vi "Global_SNK3_HF.vi"() -> ()   [LabVIEW 2017]
uses:
  Control_EU/UNDT_ClusterPackRevers (Type).ctl
  Control_EU/OptionPACK5.ctl
  E:/_git/LV_Unicorn/Control/unicorn_Param.ctl
  E:/_git/LV_Unicorn/Control/unicorn_conn.ctl
  E:/_git/LV_Unicorn/Control/unicorn_JSON.ctl
  E:/_git/LV_Unicorn/Control/unicorn_ParamInt.ctl
  E:/_git/LV_Unicorn/Control/unicorn_Telemetry.ctl
  E:/_git/LV_Unicorn/Control/unicorn_Table.ctl
  E:/_git/LV_Unicorn/Control/unicorn_ParamFloat.ctl
  E:/_git/LV_Unicorn/Control/AnswerUDP.ctl
  Control_EU/MeasControl.ctl
  E:/_git/LV_Unicorn/LV_Unicorn.lvlib
panel:
  in  "Tab Control":T1(tab)
  out "UDP1_packet_size":u16=652 caption="UDP0_packet_size"
  out "UDP1_packet_speed":dbl=652.0 caption="UDP1 packet size [Mbit/s]"
  out "UDP0_packet_speed":dbl=652.0 caption="UDP0 packet size [Mbit/s]"
  out "UDP0_EnquOverflow":bool
  out "UDP1_EnquOverflow":bool
  out "UDP0_total_size":u16=652 caption="UDP0_packet_size"
  out "UDP1_packet_nuber":u32=1995311 caption="UDP0_packet_nuber"
  out "UDP1_LostPack":u32 caption="UDP0__lost_pack"
  out "UDP1_iter_cnt":i32=7055 caption="UDP0_iter_count"
  in  "IndEnqu":enum16{"NoEnqu", "LossyEnqu", "Enqu"}(ring)=enum."Enqu"
  in  "LossyEnq":bool=TRUE
  out "UDP0":string
  out "UDP0_PackEnd_bad":u32
  out "UDP0_CRC8_bad":u32
  out "UDP0_LostPack":u32 caption="UDP0__lost_pack"
  out "UDP0_packet_size":u16=652
  out "UDP0_packet_nuber":u32=1995311
  out "UDP0_length":i32=2052
  out "UDP0_Reserv":u8
  out "UDP0_offset":i32
  out "UDP0_AscanLostPack":u32
  out "UDP0_address":u32=3232235999 format="%x"
  out "UDP0_port":u16=1555
  out "UDP0_timeout":i32=1000
  out "UDP0_iter_count":i32=7055
  in  "UDP_buf_size":i32=4000000
  in  "rx_port_0":u16=1556 caption="Порт приемника 2"
  in  "rx_port_1":u16=1557 caption="Порт приемника 1"
  in  "#UDP_pack":u32=1 min=1 max=100
  out "#el_queue":i32
  out "UNDT_Cl1":T2={"PacketCounter"=998360, "Gain Coeff"=0.0, "SamplingInterval"=2e-08, "Lose Packet"=8, "EncodersParam2"=0, "EncodersParam1"=0, "Reserve 1"=0, "Mux TX/RX"=0, "ScanDelay"=0, "CRC 8"=86, "ScanDuration"=500, "N chanel"=0, "GlobalTime2"=63660000, "GlobalTime1"=11423, "N tick"=0, "Ncycle"=15329, "FrameFormatVersion"=1, "MagicWord"=305419896, "Overload"=FALSE} {"Gain Coeff" format="%_5e"; "Reserve 1" format="%02x"; "Mux TX/RX" format="%02x"; "ScanDelay" format="%02x"; "SamplingInterval" format="%_3e"; "Lose Packet" format="%08x"; "EncodersParam2" format="%016x"; "EncodersParam1" format="%016x"; "CRC 8" format="%02x"; "N chanel" format="%02x"; "N tick" format="%02x"; "FrameFormatVersion" format="%02x"; "MagicWord" format="%.0x"}
  out "UNDT_Cl0":T2={"PacketCounter"=998360, "Gain Coeff"=0.0, "SamplingInterval"=2e-08, "Lose Packet"=8, "EncodersParam2"=0, "EncodersParam1"=0, "Reserve 1"=0, "Mux TX/RX"=0, "ScanDelay"=0, "CRC 8"=86, "ScanDuration"=500, "N chanel"=0, "GlobalTime2"=63660000, "GlobalTime1"=11423, "N tick"=0, "Ncycle"=15329, "FrameFormatVersion"=1, "MagicWord"=305419896, "Overload"=FALSE} {"Gain Coeff" format="%_5e"; "Reserve 1" format="%02x"; "Mux TX/RX" format="%02x"; "ScanDelay" format="%02x"; "SamplingInterval" format="%_3e"; "Lose Packet" format="%08x"; "EncodersParam2" format="%016x"; "EncodersParam1" format="%016x"; "CRC 8" format="%02x"; "N chanel" format="%02x"; "N tick" format="%02x"; "FrameFormatVersion" format="%02x"; "MagicWord" format="%.0x"}
  in  "UDP0_EnbLog":bool
  in  "SUdpAnswer":T3
  in  "paramUnicorn":T4={"conParam"={"ReadIntParam"=TRUE, "ReadDescrParam"=FALSE, "ReadFloatParam"=TRUE, "debug"=FALSE, "ReadJSON"=TRUE, "IP_address"="192.168.1.216", "N_attempts"=3, "type_con"=enum."TCP", "MB_address"=1, "VISA"="COM1", "connection ID"=refnum, "nameDevices"="", "timeout"=500, "port"=2000, "type_version"="0F0C0001", "baud_rate"=115200, "VersionControl"=TRUE, "TCP_conn"=FALSE, "WindowSize"=400}, "Param"={"NumParam"={"NTelem"=201, "NInt"=16, "NFloat"=10, "NTable"=2}, "ParamInt"=[], "Telemetry"=[], "Table"=[], "ParamFloat"=[]}}
  in  "reqTypeVer":i32=252444676 format="%08x"
  out "IP_PC":string="192.168.1.99" caption="IP адрес ПК"
  out "JSONStr":string="{ \"UUID\": true, \"Reset\": false, \"Enums\": [ { \"ID\": \"Enum_AlarmCompMode\", \"Name\": \"Alarm comparison mode\", \"Desc\": \"\", \"Values\": [ { \"Name\": \"XY\", \"Value\": 0, \"Desc\": \"Available for rectangular and sector zones\" }, { \"Name\": \"AT\", \"Value\": 1, \"Desc\": \"Available for measurement zone\" }, { \"Name\": \"XT\", \"Value\": 2, \"Desc\": \"Available for measurement zone\" }, { \"Name\": \"YT\", \"Value\": 3, \"Desc\": \"Available for measurement zone\" } ] }, { \"ID\": \"Enum_AlarmZonesMode\", \"Name\": \"Alarm zones mode\", \"Desc\": \"\", \"Values\": [ { \"Name\": \"off\", \"Value\": 0, \"Desc\": \"\" }, { \"Name\": \"Rectangle\", \"Value\": 1, \"Desc\": \"\" }, { \"Name\": \"sector\", \"Value\": 2, \"Desc\": \"\" }, { \"Name\": \"measurement\", \"Value\": 3, \"Desc\": \"\" } ] }, { \"ID\": \"Enum_AlarmLEDMode\", \"Name\": \"Alarm LED mode\", \"Desc\": \"\", \"Values\": [ { \"Name\": \"off\", \"Value\": 0, \"Desc\": \"LED is always off\" }, { \"Name\": \"On\", \"Value\": 1, \"Desc\": \"LED is always on\" }, { \"Name\": \"Zone1\", \"Value\": 2, \"Desc\": \"LED is on if zone 1\" }, { \"Name\": \"Zone2\", \"Value\": 3, \"Desc\": \"LED is on if zone 2\" }, { \"Name\": \"Zone3\", \"Value\": 4, \"Desc\": \"LED is on if zone 3\" }, { \"Name\": \"Zone12\", \"Value\": 5, \"Desc\": \"LED is on if zone 1 or 2\" }, { \"Name\": \"Zone13\", \"Value\": 6, \"Desc\": \"LED is on if zone 1 or 3\" }, { \"Name\": \"Zone23\", \"Value\": 7, \"Desc\": \"LED is on if zone 2 or 3\" }, { \"Name\": \"Zone123\", \"Value\": 8, \"Desc\": \"LED is on if zone 1 or 2 or 3\" } ] }, { \"ID\": \"Enum_ModeWork\", \"Name\": \"Device operation mode\", \"Desc\": \"\", \"Values\": [ { \"Name\": \"Ошибка\", \"Value\": -1, \"Desc\": \"\" }, { \"Name\": \"Конфигурирование\", \"Value\": 0, \"Desc\": \"\" }, { \"Name\": \"Сканирование\", \"Value\": 1, \"Desc\": \"\" }, { \"Name\": \"Самотестирование\", \"Value\": 2, \"Desc\": \"\" } ] }, { \"ID\": \"OnOffEnum\", \"Name\": \"On-off enum\", \"Num\": 0, \"Values\": [ { \"Name\": \"Выключено\", \"Value\": 0 }, { \"Name\": \"Включено\", \"Value\": 1 } ] }, { \"ID\": \"InvNoInvEnum\", \"Name\": \"Invert-Noinvert enum\", \"Num\": 0, \"Values\": [ { \"Name\": \"Не инвертирован\", \"Value\": 0 }, { \"Name\": \"Интерирован\", \"Value\": 1 } ] }, { \"ID\": \"Enum_SyncMode\", \"Name\": \"Режим работы узла синхронизации \", \"Desc\": \"\", \"Values\": [ { \"Name\": \"Таймер\", \"Value\": 1, \"Desc\": \"\" }, { \"Name\": \"Энкодер\", \"Value\": 2, \"Desc\": \"\" }, { \"Name\": \"Импульс\", \"Value\": 3, \"Desc\": \"\" } ] }, { \"ID\": \"Enum_LPFilter\", \"Name\": \"ФНЧ приемников\", \"Desc\": \"\", \"Values\": [ { \"Name\": \"14\", \"Value\": 0, \"Desc\": \"\" }, { \"Name\": \"10\", \"Value\": 1, \"Desc\": \"\" }, { \"Name\": \"7,5\", \"Value\": 2, \"Desc\": \"\" }, { \"Name\": \"Выключен\", \"Value\": 3, \"Desc\": \"\" } ] }, { \"ID\": \"Enum_HPFilter\", \"Name\": \"ФВЧ приемников\", \"Desc\": \"\", \"Values\": [ { \"Name\": \"Выключен\", \"Value\": 0, \"Desc\": \"\" }, { \"Name\": \"1\", \"Value\": 1, \"Desc\": \"\" }, { \"Name\": \"2\", \"Value\": 2, \"Desc\": \"\" } ] }, { \"ID\": \"Enum_PatternMode\", \"Name\": \"Тестирование цифрового интерфейса АЦП\", \"Desc\": \"\", \"Values\": [ { \"Name\": \"No pattern\", \"Value\": 0, \"Desc\": \"\" }, { \"Name\": \"Sync\", \"Value\": 1, \"Desc\": \"\" }, { \"Name\": \"Deskew\", \"Value\": 2, \"Desc\": \"\" }, { \"Name\": \"Custom\", \"Value\": 3, \"Desc\": \"\" }, { \"Name\": \"All 1s\", \"Value\": 4, \"Desc\": \"\" }, { \"Name\": \"Toggle\", \"Value\": 5, \"Desc\": \"\" }, { \"Name\": \"All 0s\", \"Value\": 6, \"Desc\": \"\" }, { \"Name\": \"Ramp\", \"Value\": 7, \"Desc\": \"\" } ] }, { \"ID\": \"Enum_PulserLevel\", \"Name\": \"Амплитуда импульсов возбуждения ГИ\", \"Desc\": \"\", \"Values\": [ { \"Name\": \"20\", \"Value\": 0, \"Desc\": \"\" }, { \"Name\": \"40\", \"Value\": 1, \"Desc\": \"\" }, { \"Name\": \"60\", \"Value\": 2, \"Desc\": \"\" }, { \"Name\": \"80\", \"Value\": 3, \"Desc\": \"\" }, { \"Name\": \"100\", \"Value\": 4, \"Desc\": \"\" }, { \"Name\": \"120\", \"Value\": 5, \"Desc\": \"\" }, { \"Name\": \"140\", \"Value\": 6, \"Desc\": \"\" }, { \"Name\": \"160\", \"Value\": 7, \"Desc\": \"\" }, { \"Name\": \"180\", \"Value\": 8, \"Desc\": \"\" }, { \"Name\": \"200\", \"Value\": 9, \"Desc\": \"\" } ] }, { \"ID\": \"DACParamEnum\", \"Name\": \"Параметр, определяющий коэффициента усиления приемников \", \"Values\": [ { \"Name\": \"Коэф. усил. (дБ)\", \"Value\": 0 }, { \"Name\": \"Вых. ЦАП (10 бит)\", \"Value\": 1 }, { \"Name\": \"Вых. ЦАП (8 бит)\", \"Value\": 1 } ] } ], \"ParamInt\": [ { \"ID\": \"ModeWork\", \"Num\": 0, \"Name\": \"Режим работы\", \"Type\": \"enum\", \"Enum\": \"Enum_ModeWork\", \"Desc\": \"\", \"Unit\": \"\", \"Access\": \"ro\" }, { \"ID\": \"CCEnable\", \"Num\": 1, \"Name\": \"Режим сканирования\", \"Type\": \"enum\", \"Enum\": \"OnOffEnum\", \"Desc\": \"Включение режима выполнения циклов сканирования\", \"Unit\": \"\", \"Access\": \"rw\" }, { \"ID\": \"CCTicksCount\", \"Num\": 2, \"Name\": \"Количество тактов\", \"Type\": \"Regular\", \"Desc\": \"Количество тактов выполняемых в каждом цикле при включении режима сканирования\", \"Unit\": \"\", \"Min\": 1, \"Max\": 32, \"FormatStr\": \"%d\", \"Access\": \"rw\" }, { \"ID\": \"LPFilter\", \"Num\": 3, \"Name\": \"ФНЧ приемников\", \"Type\": \"enum\", \"Enum\": \"Enum_LPFilter\", \"Desc\": \"Частота среза фильтра низких частот приемников сигналов элементов ФЛ\", \"Unit\": \"МГц\", \"Access\": \"rw\" }, { \"ID\": \"HPFilter\", \"Num\": 4, \"Name\": \"ФВЧ приемников\", \"Type\": \"Regular\", \"Min\": 0, \"Max\": 10, \"FormatStr\": \"%d\", \"Desc\": \"Параметр определяющий частоту среза фильтра высоких частот приемников сигналов элементов ФЛ \", \"Unit\": \"\", \"Access\": \"rw\" }, { \"ID\": \"TestTickNum\", \"Num\": 5, \"Name\": \"Номер такта для тестового захвата\", \"Desc\": \"Номер такта для выполнения тестирования настроек выбранного такта \", \"Unit\": \"\", \"Min\": 1, \"Max\": 32, \"FormatStr\": \"%d\", \"Access\": \"rw\" }, { \"ID\": \"Pulser1Level\", \"Num\": 6, \"Name\": \"Амплитуда импульсов возбуждения ГИ №1 для каналов 1…8\", \"Type\": \"enum\", \"Enum\": \"Enum_PulserLevel\", \"Desc\": \"Амплитуда импульсов возбуждения для ПЭП с 1 по 8\", \"Unit\": \"В\", \"Access\": \"rw\" }, { \"ID\": \"Pulser2Level\", \"Num\": 7, \"Name\": \"Амплитуда импульсов возбуждения ГИ №2 для каналов 9…16\", \"Type\": \"enum\", \"Enum\": \"Enum_PulserLevel\", \"Desc\": \"Амплитуда импульсов возбуждения для ПЭП с 9 по 16\", \"Unit\": \"В\", \"Access\": \"rw\" }, { \"ID\": \"IPDefaultAddress\", \"Num\": 8, \"Name\": \"IP адрес электронного блока по умолчанию\", \"Type\": \"IPv4Addr\", \"Desc\": \"Присваивается электронному блоку если не был получен автоматически от DCHP сервера\", \"Unit\": \"IPv4\", \"Access\": \"rw\" }, { \"ID\": \"IPDefaultNetMask\", \"Num\": 9, \"Name\": \"Маска подсети\", \"Type\": \"IPv4Mask\", \"Desc\": \"Присваивается электронному блоку если не был получен автоматически от DCHP сервера\", \"Unit\": \"IPv4\", \"Access\": \"rw\" }, { \"ID\": \"IPDefaultGW\", \"Num\": 10, \"Name\": \"Основной шлюз \", \"Type\": \"IPv4Addr\", \"Desc\": \"Присваивается электронному блоку если не был получен автоматически от DCHP сервера\", \"Unit\": \"IPv4\", \"Access\": \"rw\" }, { \"ID\": \"IPCurrentAddress\", \"Num\": 11, \"Name\": \"Текущий IP адрес электронного блока\", \"Type\": \"IPv4Addr\", \"Desc\": \"Присваивается электронному блоку DCHP сервером\", \"Unit\": \"IPv4\", \"Access\": \"ro\" }, { \"ID\": \"IPAddressUDP\", \"Num\": 12, \"Name\": \"IP адрес для передачи UDP пакетов\", \"Type\": \"IPv4Addr\", \"Desc\": \"IP адрес на который будут отправляется информационные UDP пакеты\", \"Unit\": \"IPv4\", \"Access\": \"rw\" }, { \"ID\": \"Port1UDP\", \"Num\": 13, \"Name\": \"Порт для передачи UDP пакетов от ГИ №1, каналы 1…8\", \"Type\": \"Regular\", \"Desc\": \"Порт, на который будут отправляется информационные UDP пакеты от ГИ №1, каналы 1…8\", \"Unit\": \"\", \"Min\": 0, \"Max\": 65535, \"FormatStr\": \"%d\", \"Access\": \"rw\" }, { \"ID\": \"Port2UDP\", \"Num\": 14, \"Name\": \"Порт для передачи UDP пакетов от ГИ №2, каналы 9…16\", \"Type\": \"Regular\", \"Desc\": \"Порт, на который будут отправляется информационные UDP пакеты от ГИ №2, каналы 9…16\", \"Unit\": \"\", \"Min\": 0, \"Max\": 65535, \"FormatStr\": \"%d\", \"Access\": \"rw\" }, { \"ID\": \"IPFPGA1TypeVer\", \"Num\": 15, \"Name\": \"Тип и версия ПЛИС №1\", \"Type\": \"Regular\", \"Desc\": \"Тип и версия встроенного ПО ПЛИС платы приема\", \"Unit\": \"\", \"FormatStr\": \"0x%08x\", \"Access\": \"ro\" }, { \"ID\": \"IPFPGA1BuildTime\", \"Num\": 16, \"Name\": \"Дата сборки ПО ПЛИС №1\", \"Type\": \"DateTime\", \"Desc\": \"Дата сборки встроенного ПО ПЛИС платы приема\", \"Unit\": \"\", \"FormatStr\": \"%T\", \"Access\": \"ro\" }, { \"ID\": \"IPFPGA2TypeVer\", \"Num\": 17, \"Name\": \"Тип и версия ПЛИС №2\", \"Type\": \"Regular\", \"Desc\": \"Тип и версия встроенного ПО ПЛИС платы приема\", \"Unit\": \"\", \"FormatStr\": \"0x%08x\", \"Access\": \"ro\" }, { \"ID\": \"IPFPGA2BuildTime\", \"Num\": 18, \"Name\": \"Дата сборки ПО ПЛИС №2\", \"Type\": \"DateTime\", \"Desc\": \"Дата сборки встроенного ПО ПЛИС платы приема\", \"Unit\": \"\", \"FormatStr\": \"%T\", \"Access\": \"ro\" }, { \"ID\": \"IPADCMonMCUBuildTime\", \"Num\": 19, \"Name\": \"Дата сборки ПО МК мониторинга\", \"Type\": \"DateTime\", \"Desc\": \"Дата сборки ПО МК мониторинга платы приема\", \"Unit\": \"\", \"FormatStr\": \"%T\", \"Access\": \"ro\" }, { \"ID\": \"IPPMD2MCUBuildTime\", \"Num\": 20, \"Name\": \"Дата сборки ПО МК мониторинга ИП D2\", \"Type\": \"DateTime\", \"Desc\": \"Дата сборки ПО МК мониторинга платы источника питания D2\", \"Unit\": \"\", \"FormatStr\": \"%T\", \"Access\": \"ro\" }, { \"ID\": \"IPPMD4MCUBuildTime\", \"Num\": 21, \"Name\": \"Дата сборки ПО МК мониторинга ИП D6\", \"Type\": \"DateTime\", \"Desc\": \"Дата сборки ПО МК мониторинга платы источника питания D6\", \"Unit\": \"\", \"FormatStr\": \"%T\", \"Access\": \"ro\" }, { \"ID\": \"IPSaveParem\", \"Num\": 22, \"Name\": \"Сохранение параметров\", \"Type\": \"bool\", \"Desc\": \"Сохранение параметров в энергонезависимую память\", \"Unit\": \"\", \"FormatStr\": \"\", \"Access\": \"rw\" }, { \"ID\": \"IPSyncMode\", \"Num\": 23, \"Name\": \"Режим работы узла синхронизации \", \"Type\": \"enum\", \"Enum\": \"Enum_SyncMode\", \"Desc\": \"Режим работы узла синхронизации \", \"Access\": \"rw\" }, { \"ID\": \"IPTimerSyncInt\", \"Num\": 24, \"Name\": \"Интервал времени запуска выполнения цикла в режиме «Таймер»\", \"Type\": \"Regular\", \"Desc\": \"-\", \"Unit\": \"мкс\", \"Min\": 1000, \"Max\": 1000000, \"FormatStr\": \"%d\", \"Access\": \"rw\" }, { \"ID\": \"IPEncoder2En\", \"Num\": 25, \"Name\": \"Разрешение работы энкодера 2\", \"Type\": \"enum\", \"Desc\": \"\", \"Enum\": \"OnOffEnum\", \"Access\": \"rw\" }, { \"ID\": \"IPEncoder1En\", \"Num\": 26, \"Name\": \"Разрешение работы энкодера 1\", \"Type\": \"enum\", \"Desc\": \"\", \"Enum\": \"OnOffEnum\", \"Access\": \"rw\" }, { \"ID\": \"IPEncoderNum\", \"Num\": 27, \"Name\": \"Номер энкодера для режима «Энкодер»\", \"Type\": \"Regular\", \"Desc\": \"\", \"Unit\": \"\", \"Min\": 1, \"Max\": 2, \"FormatStr\": \"%d\", \"Access\": \"rw\" }, { \"ID\": \"IPEncoder2ZEn\", \"Num\": 28, \"Name\": \"Энкорер 2 разрешение сброса по сигналу «Z»\", \"Type\": \"enum\", \"Desc\": \"\", \"Enum\": \"OnOffEnum\", \"Access\": \"rw\" }, { \"ID\": \"IPEncoder2ZInv\", \"Num\": 29, \"Name\": \"Энкорер 2 инверсия сигнала «Z»\", \"Type\": \"enum\", \"Desc\": \"\", \"Enum\": \"OnOffEnum\", \"Access\": \"rw\" }, { \"ID\": \"IPEncoder2BInv\", \"Num\": 30, \"Name\": \"Энкорер 2 инверсия сигнала «B»\", \"Type\": \"enum\", \"Desc\": \"\", \"Enum\": \"OnOffEnum\", \"Access\": \"rw\" }, { \"ID\": \"IPEncoder2AInv\", \"Num\": 31, \"Name\": \"Энкорер 2 инверсия сигнала «A»\", \"Type\": \"enum\", \"Desc\": \"\", \"Enum\": \"OnOffEnum\", \"Access\": \"rw\" }, { \"ID\": \"IPEncoder1ZEn\", \"Num\": 32, \"Name\": \"Энкорер 1 разрешение сброса по сигналу «Z»\", \"Type\": \"enum\", \"Desc\": \"\", \"Enum\": \"OnOffEnum\", \"Access\": \"rw\" }, { \"ID\": \"IPEncoder1ZInv\", \"Num\": 33, \"Name\": \"Энкорер 1 инверсия сигнала «Z»\", \"Type\": \"enum\", \"Desc\": \"\", \"Enum\": \"OnOffEnum\", \"Access\": \"rw\" }, { \"ID\": \"IPEncoder1BInv\", \"Num\": 34, \"Name\": \"Энкорер 1 инверсия сигнала «B»\", \"Type\": \"enum\", \"Desc\": \"\", \"Enum\": \"OnOffEnum\", \"Access\": \"rw\" }, { \"ID\": \"IPEncoder1AInv\", \"Num\": 35, \"Name\": \"Энкорер 1 инверсия сигнала «A»\", \"Type\": \"enum\", \"Desc\": \"\", \"Enum\": \"OnOffEnum\", \"Access\": \"rw\" }, { \"ID\": \"IPPulseCounterEn\", \"Num\": 36, \"Name\": \"Разрешение работы счетчика импульсов \", \"Type\": \"enum\", \"Desc\": \"\", \"Enum\": \"OnOffEnum\", \"Access\": \"rw\" }, { \"ID\": \"IPPulseInput\", \"Num\": 37, \"Name\": \"Вход импульса запуска для режима «Импульс»\", \"Type\": \"enum\", \"Desc\": \"\", \"Enum\": { \"ID\": \"IPPulseInputEnum\", \"Values\": [ { \"Desc\": \"Использовать сигнал со входа SY1_DIN1\", \"Name\": \"SY1_DIN1\", \"Value\": 0 }, { \"Desc\": \"Использовать сигнал со входа SY1_DIN2\", \"Name\": \"SY1_DIN2\", \"Value\": 1 }, { \"Desc\": \"Использовать сигнал со входа SY1_DIN3\", \"Name\": \"SY1_DIN3\", \"Value\": 2 }, { \"Desc\": \"Использовать сигнал со входа SY1_DIN4\", \"Name\": \"SY1_DIN4\", \"Value\": 3 }, { \"Desc\": \"Использовать сигнал со входа SY1_DIN5\", \"Name\": \"SY1_DIN5\", \"Value\": 4 }, { \"Desc\": \"Использовать сигнал со входа SY1_DIN6\", \"Name\": \"SY1_DIN6\", \"Value\": 5 } ] }, \"Access\": \"rw\" }, { \"ID\": \"IPPulseSensitivity\", \"Num\": 38, \"Name\": \"Чувствительность входа импульсов\", \"Type\": \"enum\", \"Desc\": \"\", \"Enum\": { \"ID\": \"IPPulseSensitivityEnum\", \"Values\": [ { \"Desc\": \"Резерв, счетчик не работает\", \"Name\": \"Резерв\", \"Value\": 0 }, { \"Desc\": \"по фронту импульса\", \"Name\": \"Фронт\", \"Value\": 1 }, { \"Desc\": \"по срезу импульса\", \"Name\": \"Срез\", \"Value\": 2 }, { \"Desc\": \"и по фронту и по срезу импульса\", \"Name\": \"Оба\", \"Value\": 3 } ] }, \"Access\": \"rw\" }, { \"ID\": \"IPDataEncodersParam2\", \"Num\": 39, \"Name\": \"Параметры поля «EncodersParam2»\", \"Type\": \"enum\", \"Desc\": \"\", \"Enum\": { \"ID\": \"IPDataEncodersParam2Enum\", \"Values\": [ { \"Desc\": \"Текущее значение счетчика энкодера 2\", \"Name\": \"Encoder2CurrData\", \"Value\": 0 }, { \"Desc\": \"Текущее значение счетчика импульсов\", \"Name\": \"PulseCurrData\", \"Value\": 1 } ] }, \"Access\": \"rw\" }, { \"ID\": \"IPDataEncodersParam1\", \"Num\": 40, \"Name\": \"Параметры поля «EncodersParam1»\", \"Type\": \"enum\", \"Desc\": \"\", \"Enum\": { \"ID\": \"IPDataEncodersParam1Enum\", \"Values\": [ { \"Desc\": \"Текущее значение счетчика энкодера 1\", \"Name\": \"Encoder1CurrData\", \"Value\": 0 }, { \"Desc\": \"Текущее значение счетчика импульсов\", \"Name\": \"PulseCurrData\", \"Value\": 1 } ] }, \"Access\": \"rw\" }, { \"ID\": \"IPEncoder1CurrDataH\", \"Num\": 41, \"Name\": \"Текущее значение счетчика энкодера 1 [старшие 32 разряда]\", \"Type\": \"Regular\", \"Desc\": \"\", \"Unit\": \"\", \"FormatStr\": \"0x%08x\", \"Access\": \"rw\" }, { \"ID\": \"IPEncoder1CurrDataL\", \"Num\": 42, \"Name\": \"Текущее значение счетчика энкодера 1 [младшие 32 разряда]\", \"Type\": \"Regular\", \"Desc\": \"\", \"Unit\": \"\", \"FormatStr\": \"0x%08x\", \"Access\": \"rw\" }, { \"ID\": \"IPEncoder2CurrDataH\", \"Num\": 43, \"Name\": \"Текущее значение счетчика энкодера 2 [старшие 32 разряда]\", \"Type\": \"Regular\", \"Desc\": \"\", \"Unit\": \"\", \"FormatStr\": \"0x%08x\", \"Access\": \"rw\" }, { \"ID\": \"IPEncoder2CurrDataL\", \"Num\": 44, \"Name\": \"Текущее значение счетчика энкодера 2 [младшие 32 разряда]\", \"Type\": \"Regular\", \"Desc\": \"\", \"Unit\": \"\", \"FormatStr\": \"0x%08x\", \"Access\": \"rw\" }, { \"ID\": \"IPPulseCurrDataH\", \"Num\": 45, \"Name\": \"Текущее значение счетчика импульсов [старшие 32 разряда]\", \"Type\": \"Regular\", \"Desc\": \"\", \"Unit\": \"\", \"FormatStr\": \"0x%08x\", \"Access\": \"rw\" }, { \"ID\": \"IPPulseCurrDataL\", \"Num\": 46, \"Name\": \"Текущее значение счетчика импульсов [младшие 32 разряда] \", \"Type\": \"Regular\", \"Desc\": \"\", \"Unit\": \"\", \"FormatStr\": \"0x%08x\", \"Access\": \"rw\" }, { \"ID\": \"IPNumOfRuns\", \"Num\": 47, \"Name\": \"Текущее значение счетчика количества запусков цикла\", \"Type\": \"Regular\", \"Desc\": \"\", \"Unit\": \"\", \"FormatStr\": \"%d\", \"Access\": \"ro\" }, { \"ID\": \"IPEncoderSyncH\", \"Num\": 48, \"Name\": \"Величина «К» [старшие 32 разряда]\", \"Type\": \"Regular\", \"Desc\": \"\", \"Unit\": \"\", \"FormatStr\": \"0x%08x\", \"Access\": \"rw\" }, { \"ID\": \"IPEncoderSyncL\", \"Num\": 49, \"Name\": \"Величина «К» [младшие 32 разряда]\", \"Type\": \"Regular\", \"Desc\": \"\", \"Unit\": \"\", \"FormatStr\": \"0x%08x\", \"Access\": \"rw\" }, { \"ID\": \"IPEncoder1ScalingFactor\", \"Num\": 50, \"Name\": \"Масштабный коэффициент для Энкодера 1\", \"Type\": \"Regular\", \"Desc\": \"\", \"Unit\": \"нм/имп\", \"FormatStr\": \"%d\", \"Access\": \"rw\" }, { \"ID\": \"IPEncoder2ScalingFactor\", \"Num\": 51, \"Name\": \"Масштабный коэффициент для Энкодера 2\", \"Type\": \"Regular\", \"Desc\": \"\", \"Unit\": \"нм/имп\", \"FormatStr\": \"%d\", \"Access\": \"rw\" }, { \"ID\": \"IPPulseScalingFactor\", \"Num\": 52, \"Name\": \"Масштабный коэффициент для режима «Импульс»\", \"Type\": \"Regular\", \"Desc\": \"\", \"Unit\": \"нм/имп\", \"FormatStr\": \"%d\", \"Access\": \"rw\" }, { \"ID\": \"IPCalReceiveDelay\", \"Num\": 53, \"Name\": \"Сдвиг времени начала приема\", \"Type\": \"Regular\", \"Desc\": \"\", \"Unit\": \"имп\", \"FormatStr\": \"%d\", \"Access\": \"rw\" }, { \"ID\": \"IPReceiverStaticGainParam\", \"Num\": 54, \"Name\": \"Параметр, определяющий коэффициента усиления приемников\", \"Type\": \"enum\", \"Enum\": \"DACParamEnum\", \"Desc\": \"Определяет какой из табличных параметров будет отвечать за установку коэффициента усиления приемника\", \"Unit\": \"\", \"Access\": \"rw\" }, { \"ID\": \"IPServiceCode\", \"Num\": 55, \"Name\": \"Сервисный код\", \"Type\": \"Regular\", \"Desc\": \"\", \"FormatStr\": \"%d\", \"Access\": \"rw\" }, { \"ID\": \"IPEn50OmOut\", \"Num\": 56, \"Name\": \"Демпфирование ПЭП (50 Ом)\", \"Type\": \"enum\", \"Enum\": \"OnOffEnum\", \"Desc\": \"\", \"Unit\": \"\", \"Access\": \"rw\" }, { \"ID\": \"IPRB0MCUBuildTime\", \"Num\": 57, \"Name\": \"Дата сборки ПО МК RB №1\", \"Type\": \"DateTime\", \"Desc\": \"Дата сборки встроенного ПО МК платы приема, входы 1..8\", \"Unit\": \"\", \"FormatStr\": \"%T\", \"Access\": \"ro\" }, { \"ID\": \"IPRB1MCUBuildTime\", \"Num\": 58, \"Name\": \"Дата сборки ПО МК RB №2\", \"Type\": \"DateTime\", \"Desc\": \"Дата сборки встроенного ПО МК платы приема, входы 9..16\", \"Unit\": \"\", \"FormatStr\": \"%T\", \"Access\": \"ro\" }, { \"ID\": \"IPAFE0MCUBuildTime\", \"Num\": 59, \"Name\": \"Дата сборки ПО МК AFE №1\", \"Type\": \"DateTime\", \"Desc\": \"Дата сборки встроенного ПО МК платы коммутатора, входы 1..8\", \"Unit\": \"\", \"FormatStr\": \"%T\", \"Access\": \"ro\" }, { \"ID\": \"IPAFE1MCUBuildTime\", \"Num\": 60, \"Name\": \"Дата сборки ПО МК AFE №2\", \"Type\": \"DateTime\", \"Desc\": \"Дата сборки встроенного ПО МК платы коммутатора, входы 9..16\", \"Unit\": \"\", \"FormatStr\": \"%T\", \"Access\": \"ro\" }, { \"ID\": \"IPPAB0MCUBuildTime\", \"Num\": 61, \"Name\": \"Дата сборки ПО МК PAB №1\", \"Type\": \"DateTime\", \"Desc\": \"Дата сборки встроенного ПО МК платы усилителей мощности, входы 1..8\", \"Unit\": \"\", \"FormatStr\": \"%T\", \"Access\": \"ro\" }, { \"ID\": \"IPPAB1MCUBuildTime\", \"Num\": 62, \"Name\": \"Дата сборки ПО МК PAB №2\", \"Type\": \"DateTime\", \"Desc\": \"Дата сборки встроенного ПО МК платы усилителей мощности, входы 9..16\", \"Unit\": \"\", \"FormatStr\": \"%T\", \"Access\": \"ro\" }, { \"ID\": \"IPFPGA0ExtRAMBuffEn\", \"Num\": 63, \"Name\": \"Буферезация потока данных в SRAM для каналов 1-8\", \"Type\": \"enum\", \"Enum\": \"OnOffEnum\", \"Desc\": \"\", \"Unit\": \"\", \"Access\": \"rw\" }, { \"ID\": \"IPFPGA1ExtRAMBuffEn\", \"Num\": 64, \"Name\": \"Буферезация потока данных в SRAM для каналов 9-16\", \"Type\": \"enum\", \"Enum\": \"OnOffEnum\", \"Desc\": \"\", \"Unit\": \"\", \"Access\": \"rw\" }, { \"ID\": \"IPFPGAExtRAMTest\", \"Num\": 65, \"Name\": \"Тестирование SRAM\", \"Type\": \"enum\", \"Desc\": \"\", \"Enum\": { \"ID\": \"IPFPGAExtRAMTestEnum\", \"Values\": [ { \"Desc\": \"\", \"Name\": \"Не выполняется\", \"Value\": 0 }, { \"Desc\": \"\", \"Name\": \"Выполняется\", \"Value\": 1 } ] }, \"Access\": \"rw\" }, { \"ID\": \"IPFPGAExtRAMTestError\", \"Num\": 66, \"Name\": \"Ошибки тестирование SRAM\", \"Type\": \"Regular\", \"Desc\": \"\", \"FormatStr\": \"0x%08x\", \"Access\": \"ro\" }, { \"ID\": \"IPSerialNumber\", \"Num\": 67, \"Name\": \"Заводской номер\", \"Type\": \"Regular\", \"Desc\": \"\", \"FormatStr\": \"%d\", \"Access\": \"rw\" }, { \"ID\": \"IPAddPulseDelayP\", \"Num\": 68, \"Name\": \"AddPulseDelayP\", \"Type\": \"Regular\", \"Desc\": \"\", \"FormatStr\": \"%d\", \"Access\": \"rw\" }, { \"ID\": \"IPAddPulseDurationP\", \"Num\": 69, \"Name\": \"AddPulseDurationP\", \"Type\": \"Regular\", \"Desc\": \"\", \"FormatStr\": \"%d\", \"Access\": \"rw\" }, { \"ID\": \"IPAddPulseDelayN\", \"Num\": 70, \"Name\": \"AddPulseDelayN\", \"Type\": \"Regular\", \"Desc\": \"\", \"FormatStr\": \"%d\", \"Access\": \"rw\" }, { \"ID\": \"IPAddPulseDurationN\", \"Num\": 71, \"Name\": \"AddPulseDurationN\", \"Type\": \"Regular\", \"Desc\": \"\", \"FormatStr\": \"%d\", \"Access\": \"rw\" }, { \"ID\": \"IPPAB_SellHVFinePL0\", \"Num\": 72, \"Name\": \"PAB_SellHVFinePL0\", \"Type\": \"Regular\", \"Desc\": \"\", \"FormatStr\": \"%d\", \"Access\": \"rw\" }, { \"ID\": \"IPPAB_SellHVFinePL1\", \"Num\": 73, \"Name\": \"PAB_SellHVFinePL1\", \"Type\": \"Regular\", \"Desc\": \"\", \"FormatStr\": \"%d\", \"Access\": \"rw\" }, { \"ID\": \"IPSyncPowerMode\", \"Num\": 74, \"Name\": \"SyncPowerMode\", \"Type\": \"enum\", \"Enum\": \"OnOffEnum\", \"Desc\": \"\", \"FormatStr\": \"%d\", \"Access\": \"rw\" }, { \"ID\": \"IPStatus_HF_EU\", \"Num\": 75, \"Name\": \"Status_HF_EU\", \"Type\": \"Regular\", \"Desc\": \"\", \"FormatStr\": \"0x%08x\", \"Access\": \"rw\" }, { \"ID\": \"IPNumDataInFIFO_PL0\", \"Num\": 76, \"Name\": \"NumDataInFIFO_PL0\", \"Type\": \"Regular\", \"Desc\": \"\", \"FormatStr\": \"%d\", \"Access\": \"rw\" }, { \"ID\": \"IPNumDataInFIFO_PL1\", \"Num\": 77, \"Name\": \"NumDataInFIFO_PL1\", \"Type\": \"Regular\", \"Desc\": \"\", \"FormatStr\": \"%d\", \"Access\": \"rw\" } ], \"ParamFloat\": [ { \"ID\": \"FPGainSlopePL0\", \"Num\": 0, \"Name\": \"GainSlopePL0\", \"Type\": \"Regular\", \"Desc\": \"Частота среза\", \"Unit\": \"\", \"Min\": -100.0, \"Max\": -100.0, \"FormatStr\": \"%f\", \"Access\": \"rw\" }, { \"ID\": \"FPGainSlopePL1\", \"Num\": 1, \"Name\": \"GainSlopePL1\", \"Type\": \"Regular\", \"Desc\": \"Частота среза\", \"Unit\": \"\", \"Min\": -100.0, \"Max\": -100.0, \"FormatStr\": \"%f\", \"Access\": \"rw\" }, { \"ID\": \"FPGainOfsetPL0\", \"Num\": 2, \"Name\": \"GainOfsetPL0\", \"Type\": \"Regular\", \"Desc\": \"Частота среза\", \"Unit\": \"\", \"Min\": -100.0, \"Max\": -100.0, \"FormatStr\": \"%f\", \"Access\": \"rw\" }, { \"ID\": \"FPGainOfsetPL1\", \"Num\": 3, \"Name\": \"GainOfsetPL1\", \"Type\": \"Regular\", \"Desc\": \"Частота среза\", \"Unit\": \"\", \"Min\": -100.0, \"Max\": -100.0, \"FormatStr\": \"%f\", \"Access\": \"rw\" }, { \"ID\": \"FPGainSlopeSecPL0\", \"Num\": 4, \"Name\": \"GainSlopeSecPL0\", \"Type\": \"Regular\", \"Desc\": \"Частота среза\", \"Unit\": \"\", \"Min\": -100.0, \"Max\": -100.0, \"FormatStr\": \"%f\", \"Access\": \"rw\" }, { \"ID\": \"FPGainSlopeSecPL1\", \"Num\": 5, \"Name\": \"GainSlopeSecPL1\", \"Type\": \"Regular\", \"Desc\": \"Частота среза\", \"Unit\": \"\", \"Min\": -100.0, \"Max\": -100.0, \"FormatStr\": \"%f\", \"Access\": \"rw\" }, { \"ID\": \"FPGainOfsetSecPL0\", \"Num\": 6, \"Name\": \"GainOffsetSecPL0\", \"Type\": \"Regular\", \"Desc\": \"Частота среза\", \"Unit\": \"\", \"Min\": -100.0, \"Max\": -100.0, \"FormatStr\": \"%f\", \"Access\": \"rw\" }, { \"ID\": \"FPGainOfsetSecPL1\", \"Num\": 7, \"Name\": \"GainOffsetSecPL1\", \"Type\": \"Regular\", \"Desc\": \"Частота среза\", \"Unit\": \"\", \"Min\": -100.0, \"Max\": -100.0, \"FormatStr\": \"%f\", \"Access\": \"rw\" } ], \"Telemetry\": [ { \"ID\": \"CoreUptime\", \"Num\": 0, \"Name\": \"Core uptime\", \"Desc\": \"\", \"Unit\": \"s\", \"FormatStr\": \"%.1f\" }, { \"ID\": \"EP2C8time1\", \"Num\": 1, \"Name\": \"FPGA №1 uptime\", \"Desc\": \"\", \"Unit\": \"s\", \"FormatStr\": \"%.1f\" }, { \"ID\": \"EP2C8time2\", \"Num\": 2, \"Name\": \"FPGA №2 uptime\", \"Desc\": \"\", \"Unit\": \"s\", \"FormatStr\": \"%.1f\" }, { \"ID\": \"TelStatusHF_EU\", \"Num\": 3, \"Name\": \"TelStatusHF_EU\", \"Desc\": \"\", \"Unit\": \"\", \"Min\": -0.01, \"Max\": 0.01, \"FormatStr\": \"%.0f\" }, { \"ID\": \"TelEncoder1CurrData\", \"Num\": 4, \"Name\": \"Энкодер №1\", \"Desc\": \"Текущее значение счетчика энкодера №1 модуля синхронизации\", \"Unit\": \"мкм\", \"FormatStr\": \"%.0f\" }, { \"ID\": \"TelPulseCurrData\", \"Num\": 5, \"Name\": \"Счетчик импыльсов\", \"Desc\": \"Текущее значение счетчика импульсов модуля синхронизации\", \"Unit\": \"мкм\", \"FormatStr\": \"%.0f\" }, { \"ID\": \"TelEncoderParam1\", \"Num\": 6, \"Name\": \"EncoderParam1\", \"Desc\": \"Значение поля «EncoderParam1» пакетов потока передачи данных\", \"Unit\": \"мкм\", \"FormatStr\": \"%.0f\" }, { \"ID\": \"TelEncoderParam2\", \"Num\": 7, \"Name\": \"EncoderParam2\", \"Desc\": \"Значение поля «EncoderParam2» пакетов потока передачи данных\", \"Unit\": \"мкм\", \"FormatStr\": \"%.0f\" }, { \"ID\": \"Tel33VDMON_G_min\", \"Num\": 8, \"Name\": \"Tel33VDMON_G_min\", \"Desc\": \"\", \"Unit\": \"В\", \"FormatStr\": \"%.3f\" }, { \"ID\": \"Tel33VDMON_G_avg\", \"Num\": 9, \"Name\": \"Tel33VDMON_G_avg\", \"Desc\": \"\", \"Unit\": \"В\", \"FormatStr\": \"%.3f\" }, { \"ID\": \"Tel33VDMON_G_max\", \"Num\": 10, \"Name\": \"Tel33VDMON_G_max\", \"Desc\": \"\", \"Unit\": \"В\", \"FormatStr\": \"%.3f\" }, { \"ID\": \"TelPMD2TempSensor\", \"Num\": 11, \"Name\": \"TelPMD2TempSensor\", \"Desc\": \"\", \"Unit\": \"°C\", \"Min\": 10.0, \"Max\": 80.0, \"FormatStr\": \"%.1f\" }, { \"ID\": \"TelPMD2TempDS18B20\", \"Num\": 12, \"Name\": \"TelPMD2TempDS18B20\", \"Desc\": \"\", \"Unit\": \"°C\", \"Min\": 10.0, \"Max\": 80.0, \"FormatStr\": \"%.1f\" }, { \"ID\": \"TelPMD6TempSensor\", \"Num\": 13, \"Name\": \"TelPMD6TempSensor\", \"Desc\": \"\", \"Unit\": \"°C\", \"Min\": 10.0, \"Max\": 80.0, \"FormatStr\": \"%.1f\" }, { \"ID\": \"TelPMD6TempDS18B20\", \"Num\": 14, \"Name\": \"TelPMD6TempDS18B20\", \"Desc\": \"\", \"Unit\": \"°C\", \"Min\": 10.0, \"Max\": 80.0, \"FormatStr\": \"%.1f\" }, { \"ID\": \"rb0_TempSensor\", \"Num\": 15, \"Name\": \"rb0_TempSensor\", \"Desc\": \"\", \"Unit\": \"°C\", \"Min\": 10.0, \"Max\": 80.0, \"FormatStr\": \"%.1f\" }, { \"ID\": \"rb1_TempSensor\", \"Num\": 16, \"Name\": \"rb1_TempSensor\", \"Desc\": \"\", \"Unit\": \"°C\", \"Min\": 10.0, \"Max\": 80.0, \"FormatStr\": \"%.1f\" }, { \"ID\": \"afe0_TempSensor\", \"Num\": 17, \"Name\": \"afe0_TempSensor\", \"Desc\": \"\", \"Unit\": \"°C\", \"Min\": 10.0, \"Max\": 80.0, \"FormatStr\": \"%.1f\" }, { \"ID\": \"afe0_TempDS18B20\", \"Num\": 18, \"Name\": \"afe0_TempDS18B20\", \"Desc\": \"\", \"Unit\": \"°C\", \"Min\": 10.0, \"Max\": 80.0, \"FormatStr\": \"%.1f\" }, { \"ID\": \"afe1_TempSensor\", \"Num\": 19, \"Name\": \"afe1_TempSensor\", \"Desc\": \"\", \"Unit\": \"°C\", \"Min\": 10.0, \"Max\": 80.0, \"FormatStr\": \"%.1f\" }, { \"ID\": \"afe1_TempDS18B20\", \"Num\": 20, \"Name\": \"afe1_TempDS18B20\", \"Desc\": \"\", \"Unit\": \"°C\", \"Min\": 10.0, \"Max\": 80.0, \"FormatStr\": \"%.1f\" }, { \"ID\": \"pab0_TempSensor\", \"Num\": 21, \"Name\": \"pab0_TempSensor\", \"Desc\": \"\", \"Unit\": \"°C\", \"Min\": 10.0, \"Max\": 80.0, \"FormatStr\": \"%.1f\" }, { \"ID\": \"pab0_TempDS18B20\", \"Num\": 22, \"Name\": \"pab0_TempDS18B20\", \"Desc\": \"\", \"Unit\": \"°C\", \"Min\": 10.0, \"Max\": 80.0, \"FormatStr\": \"%.1f\" }, { \"ID\": \"pab1_TempSensor\", \"Num\": 23, \"Name\": \"pab1_TempSensor\", \"Desc\": \"\", \"Unit\": \"°C\", \"Min\": 10.0, \"Max\": 80.0, \"FormatStr\": \"%.1f\" }, { \"ID\": \"pab1_TempDS18B20\", \"Num\": 24, \"Name\": \"pab1_TempDS18B20\", \"Desc\": \"\", \"Unit\": \"°C\", \"Min\": 10.0, \"Max\": 80.0, \"FormatStr\": \"%.1f\" }, { \"ID\": \"TelPMD2CInMin\", \"Num\": 25, \"Name\": \"TelPMD2CInMin\", \"Desc\": \"\", \"Unit\": \"A\", \"Min\": 0.1, \"Max\": 3.15, \"FormatStr\": \"%.3f\" }, { \"ID\": \"TelPMD2CInAVG\", \"Num\": 26, \"Name\": \"TelPMD2CInAVG\", \"Desc\": \"\", \"Unit\": \"A\", \"Min\": 0.1, \"Max\": 3.15, \"FormatStr\": \"%.3f\" }, { \"ID\": \"TelPMD2CInMax\", \"Num\": 27, \"Name\": \"TelPMD2CInMax\", \"Desc\": \"\", \"Unit\": \"A\", \"Min\": 0.1, \"Max\": 3.15, \"FormatStr\": \"%.3f\" }, { \"ID\": \"TelPMD2VInMin\", \"Num\": 28, \"Name\": \"TelPMD2VInMin\", \"Desc\": \"\", \"Unit\": \"V\", \"Min\": 10.5, \"Max\": 14.0, \"FormatStr\": \"%.3f\" }, { \"ID\": \"TelPMD2VInAVG\", \"Num\": 29, \"Name\": \"TelPMD2VInAVG\", \"Desc\": \"\", \"Unit\": \"V\", \"Min\": 10.5, \"Max\": 14.0, \"FormatStr\": \"%.3f\" }, { \"ID\": \"TelPMD2VInMax\", \"Num\": 30, \"Name\": \"TelPMD2VInMax\", \"Desc\": \"\", \"Unit\": \"V\", \"Min\": 10.5, \"Max\": 14.0, \"FormatStr\": \"%.3f\" }, { \"ID\": \"TelPMD2PInMin\", \"Num\": 31, \"Name\": \"TelPMD2PInMin\", \"Desc\": \"\", \"Unit\": \"W\", \"Min\": 1.0, \"Max\": 30.0, \"FormatStr\": \"%.3f\" }, { \"ID\": \"TelPMD2PInAVG\", \"Num\": 32, \"Name\": \"TelPMD2PInAVG\", \"Desc\": \"\", \"Unit\": \"W\", \"Min\": 1.0, \"Max\": 30.0, \"FormatStr\": \"%.3f\" }, { \"ID\": \"TelPMD2PInMax\", \"Num\": 33, \"Name\": \"TelPMD2PInMax\", \"Desc\": \"\", \"Unit\": \"W\", \"Min\": 1.0, \"Max\": 30.0, \"FormatStr\": \"%.3f\" }, { \"ID\": \"TelPMD2ConvFreq\", \"Num\": 34, \"Name\": \"TelPMD2ConvFreq\", \"Desc\": \"\", \"Unit\": \"Hz\", \"Min\": 120.0e3, \"Max\": 135.0e3, \"FormatStr\": \"%.0f\" }, { \"ID\": \"TelPMD6Vp220VMin\", \"Num\": 35, \"Name\": \"TelPMD6Vp220VMin\", \"Desc\": \"\", \"Unit\": \"V\", \"Min\": 215.0, \"Max\": 230.0, \"FormatStr\": \"%.3f\" }, { \"ID\": \"TelPMD6Vp220VAVG\", \"Num\": 36, \"Name\": \"TelPMD6Vp220VAVG\", \"Desc\": \"\", \"Unit\": \"V\", \"Min\": 215.0, \"Max\": 230.0, \"FormatStr\": \"%.3f\" }, { \"ID\": \"TelPMD6Vp220VMax\", \"Num\": 37, \"Name\": \"TelPMD6Vp220VMax\", \"Desc\": \"\", \"Unit\": \"V\", \"Min\": 215.0, \"Max\": 230.0, \"FormatStr\": \"%.3f\" }, { \"ID\": \"TelPMD6Vp8VMin\", \"Num\": 38, \"Name\": \"TelPMD6Vp8VMin\", \"Desc\": \"\", \"Unit\": \"V\", \"Min\": 7.0, \"Max\": 9.5, \"FormatStr\": \"%.3f\" }, { \"ID\": \"TelPMD6Vp8VAVG\", \"Num\": 39, \"Name\": \"TelPMD6Vp8VAVG\", \"Desc\": \"\", \"Unit\": \"V\", \"Min\": 7.0, \"Max\": 9.5, \"FormatStr\": \"%.3f\" }, { \"ID\": \"TelPMD6Vp8VMax\", \"Num\": 40, \"Name\": \"TelPMD6Vp8VMax\", \"Desc\": \"\", \"Unit\": \"V\", \"Min\": 7.0, \"Max\": 9.5, \"FormatStr\": \"%.3f\" }, { \"ID\": \"TelPMD6Vp5VMin\", \"Num\": 41, \"Name\": \"TelPMD6Vp5VMin\", \"Desc\": \"\", \"Unit\": \"V\", \"Min\": 4.8, \"Max\": 5.3, \"FormatStr\": \"%.3f\" }, { \"ID\": \"TelPMD6Vp5VAVG\", \"Num\": 42, \"Name\": \"TelPMD6Vp5VAVG\", \"Desc\": \"\", \"Unit\": \"V\", \"Min\": 4.8, \"Max\": 5.3, \"FormatStr\": \"%.3f\" }, { \"ID\": \"TelPMD6Vp5VMax\", \"Num\": 43, \"Name\": \"TelPMD6Vp5VMax\", \"Desc\": \"\", \"Unit\": \"V\", \"Min\": 4.8, \"Max\": 5.3, \"FormatStr\": \"%.3f\" }, { \"ID\": \"TelPMD6Vp20VMin\", \"Num\": 44, \"Name\": \"TelPMD6Vp20VMin\", \"Desc\": \"\", \"Unit\": \"V\", \"Min\": 17.0, \"Max\": 19.0, \"FormatStr\": \"%.3f\" }, { \"ID\": \"TelPMD6Vp20VAVG\", \"Num\": 45, \"Name\": \"TelPMD6Vp20VAVG\", \"Desc\": \"\", \"Unit\": \"V\", \"Min\": 17.0, \"Max\": 19.0, \"FormatStr\": \"%.3f\" }, { \"ID\": \"TelPMD6Vp20VMax\", \"Num\": 46, \"Name\": \"TelPMD6Vp20VMax\", \"Desc\": \"\", \"Unit\": \"V\", \"Min\": 17.0, \"Max\": 19.0, \"FormatStr\": \"%.3f\" }, { \"ID\": \"TelPMD6Vn8VMin\", \"Num\": 47, \"Name\": \"TelPMD6Vn8VMin\", \"Desc\": \"\", \"Unit\": \"V\", \"Min\": -9.5, \"Max\": -7.0, \"FormatStr\": \"%.3f\" }, { \"ID\": \"TelPMD6Vn8VAVG\", \"Num\": 48, \"Name\": \"TelPMD6Vn8VAVG\", \"Desc\": \"\", \"Unit\": \"V\", \"Min\": -9.5, \"Max\": -7.0, \"FormatStr\": \"%.3f\" }, { \"ID\": \"TelPMD6Vn8VMax\", \"Num\": 49, \"Name\": \"TelPMD6Vn8VMax\", \"Desc\": \"\", \"Unit\": \"V\", \"Min\": -9.5, \"Max\": -7.0, \"FormatStr\": \"%.3f\" }, { \"ID\": \"TelPMD6Vn20VMin\", \"Num\": 50, \"Name\": \"TelPMD6Vn20VMin\", \"Desc\": \"\", \"Unit\": \"V\", \"Min\": -20.0, \"Max\": -17.0, \"FormatStr\": \"%.3f\" }, { \"ID\": \"TelPMD6Vn20VAVG\", \"Num\": 51, \"Name\": \"TelPMD6Vn20VAVG\", \"Desc\": \"\", \"Unit\": \"V\", \"Min\": -20.0, \"Max\": -17.0, \"FormatStr\": \"%.3f\" }, { \"ID\": \"TelPMD6Vn20VMax\", \"Num\": 52, \"Name\": \"TelPMD6Vn20VMax\", \"Desc\": \"\", \"Unit\": \"V\", \"Min\": -20.0, \"Max\": -17.0, \"FormatStr\": \"%.3f\" }, { \"ID\": \"rb0_p_1v2d_G_min\", \"Num\": 53, \"Name\": \"rb0_p_1v2d_G_min\", \"Desc\": \"\", \"Unit\": \"V\", \"Min\": 1.15, \"Max\": 1.30, \"FormatStr\": \"%.3f\" }, { \"ID\": \"rb0_p_1v2d_G_avg\", \"Num\": 54, \"Name\": \"rb0_p_1v2d_G_avg\", \"Desc\": \"\", \"Unit\": \"V\", \"Min\": 1.15, \"Max\": 1.30, \"FormatStr\": \"%.3f\" }, { \"ID\": \"rb0_p_1v2d_G_max\", \"Num\": 55, \"Name\": \"rb0_p_1v2d_G_max\", \"Desc\": \"\", \"Unit\": \"V\", \"Min\": 1.15, \"Max\": 1.30, \"FormatStr\": \"%.3f\" }, { \"ID\": \"rb0_p_1v8a_G_min\", \"Num\": 56, \"Name\": \"rb0_p_1v8a_G_min\", \"Desc\": \"\", \"Unit\": \"V\", \"Min\": 1.70, \"Max\": 1.90, \"FormatStr\": \"%.3f\" }, { \"ID\": \"rb0_p_1v8a_G_avg\", \"Num\": 57, \"Name\": \"rb0_p_1v8a_G_avg\", \"Desc\": \"\", \"Unit\": \"V\", \"Min\": 1.70, \"Max\": 1.90, \"FormatStr\": \"%.3f\" }, { \"ID\": \"rb0_p_1v8a_G_max\", \"Num\": 58, \"Name\": \"rb0_p_1v8a_G_max\", \"Desc\": \"\", \"Unit\": \"V\", \"Min\": 1.70, \"Max\": 1.90, \"FormatStr\": \"%.3f\" }, { \"ID\": \"rb0_p_3v3d_G_min\", \"Num\": 59, \"Name\": \"rb0_p_3v3d_G_min\", \"Desc\": \"\", \"Unit\": \"V\", \"Min\": 3.2, \"Max\": 3.4, \"FormatStr\": \"%.3f\" }, { \"ID\": \"rb0_p_3v3d_G_avg\", \"Num\": 60, \"Name\": \"rb0_p_3v3d_G_avg\", \"Desc\": \"\", \"Unit\": \"V\", \"Min\": 3.2, \"Max\": 3.4, \"FormatStr\": \"%.3f\" }, { \"ID\": \"rb0_p_3v3d_G_max\", \"Num\": 61, \"Name\": \"rb0_p_3v3d_G_max\", \"Desc\": \"\", \"Unit\": \"V\", \"Min\": 3.2, \"Max\": 3.4, \"FormatStr\": \"%.3f\" }, { \"ID\": \"rb0_p_5va_G_min\", \"Num\": 62, \"Name\": \"rb0_p_5va_G_min\", \"Desc\": \"\", \"Unit\": \"V\", \"Min\": 4.9, \"Max\": 5.1, \"FormatStr\": \"%.3f\" }, { \"ID\": \"rb0_p_5va_G_avg\", \"Num\": 63, \"Name\": \"rb0_p_5va_G_avg\", \"Desc\": \"\", \"Unit\": \"V\", \"Min\": 4.9, \"Max\": 5.1, \"FormatStr\": \"%.3f\" }, { \"ID\": \"rb0_p_5va_G_max\", \"Num\": 64, \"Name\": \"rb0_p_5va_G_max\", \"Desc\": \"\", \"Unit\": \"V\", \"Min\": 4.9, \"Max\": 5.1, \"FormatStr\": \"%.3f\" }, { \"ID\": \"rb1_p_1v2d_G_min\", \"Num\": 65, \"Name\": \"rb1_p_1v2d_G_min\", \"Desc\": \"\", \"Unit\": \"V\", \"Min\": 1.15, \"Max\": 1.30, \"FormatStr\": \"%.3f\" }, { \"ID\": \"rb1_p_1v2d_G_avg\", \"Num\": 66, \"Name\": \"rb1_p_1v2d_G_avg\", \"Desc\": \"\", \"Unit\": \"V\", \"Min\": 1.15, \"Max\": 1.30, \"FormatStr\": \"%.3f\" }, { \"ID\": \"rb1_p_1v2d_G_max\", \"Num\": 67, \"Name\": \"rb1_p_1v2d_G_max\", \"Desc\": \"\", \"Unit\": \"V\", \"Min\": 1.15, \"Max\": 1.30, \"FormatStr\": \"%.3f\" }, { \"ID\": \"rb1_p_1v8a_G_min\", \"Num\": 68, \"Name\": \"rb1_p_1v8a_G_min\", \"Desc\": \"\", \"Unit\": \"V\", \"Min\": 1.70, \"Max\": 1.90, \"FormatStr\": \"%.3f\" }, { \"ID\": \"rb1_p_1v8a_G_avg\", \"Num\": 69, \"Name\": \"rb1_p_1v8a_G_avg\", \"Desc\": \"\", \"Unit\": \"V\", \"Min\": 1.70, \"Max\": 1.90, \"FormatStr\": \"%.3f\" }, { \"ID\": \"rb1_p_1v8a_G_max\", \"Num\": 70, \"Name\": \"rb1_p_1v8a_G_max\", \"Desc\": \"\", \"Unit\": \"V\", \"Min\": 1.70, \"Max\": 1.90, \"FormatStr\": \"%.3f\" }, { \"ID\": \"rb1_p_3v3d_G_min\", \"Num\": 71, \"Name\": \"rb1_p_3v3d_G_min\", \"Desc\": \"\", \"Unit\": \"V\", \"Min\": 3.2, \"Max\": 3.4, \"FormatStr\": \"%.3f\" }, { \"ID\": \"rb1_p_3v3d_G_avg\", \"Num\": 72, \"Name\": \"rb1_p_3v3d_G_avg\", \"Desc\": \"\", \"Unit\": \"V\", \"Min\": 3.2, \"Max\": 3.4, \"FormatStr\": \"%.3f\" }, { \"ID\": \"rb1_p_3v3d_G_max\", \"Num\": 73, \"Name\": \"rb1_p_3v3d_G_max\", \"Desc\": \"\", \"Unit\": \"V\", \"Min\": 3.2, \"Max\": 3.4, \"FormatStr\": \"%.3f\" }, { \"ID\": \"rb1_p_5va_G_min\", \"Num\": 74, \"Name\": \"rb1_p_5va_G_min\", \"Desc\": \"\", \"Unit\": \"V\", \"Min\": 4.9, \"Max\": 5.1, \"FormatStr\": \"%.3f\" }, { \"ID\": \"rb1_p_5va_G_avg\", \"Num\": 75, \"Name\": \"rb1_p_5va_G_avg\", \"Desc\": \"\", \"Unit\": \"V\", \"Min\": 4.9, \"Max\": 5.1, \"FormatStr\": \"%.3f\" }, { \"ID\": \"rb1_p_5va_G_max\", \"Num\": 76, \"Name\": \"rb1_p_5va_G_max\", \"Desc\": \"\", \"Unit\": \"V\", \"Min\": 4.9, \"Max\": 5.1, \"FormatStr\": \"%.3f\" }, { \"ID\": \"afe0_p_20v_G_min\", \"Num\": 77, \"Name\": \"afe0_p_20v_G_min\", \"Desc\": \"\", \"Unit\": \"V\", \"Min\": 17.0, \"Max\": 19.0, \"FormatStr\": \"%.3f\" }, { \"ID\": \"afe0_p_20v_G_avg\", \"Num\": 78, \"Name\": \"afe0_p_20v_G_avg\", \"Desc\": \"\", \"Unit\": \"V\", \"Min\": 17.0, \"Max\": 19.0, \"FormatStr\": \"%.3f\" }, { \"ID\": \"afe0_p_20v_G_max\", \"Num\": 79, \"Name\": \"afe0_p_20v_G_max\", \"Desc\": \"\", \"Unit\": \"V\", \"Min\": 17.0, \"Max\": 19.0, \"FormatStr\": \"%.3f\" }, { \"ID\": \"afe0_p_8v_G_min\", \"Num\": 80, \"Name\": \"afe0_p_8v_G_min\", \"Desc\": \"\", \"Unit\": \"V\", \"Min\": 7.0, \"Max\": 9.5, \"FormatStr\": \"%.3f\" }, { \"ID\": \"afe0_p_8v_G_avg\", \"Num\": 81, \"Name\": \"afe0_p_8v_G_avg\", \"Desc\": \"\", \"Unit\": \"V\", \"Min\": 7.0, \"Max\": 9.5, \"FormatStr\": \"%.3f\" }, { \"ID\": \"afe0_p_8v_G_max\", \"Num\": 82, \"Name\": \"afe0_p_8v_G_max\", \"Desc\": \"\", \"Unit\": \"V\", \"Min\": 7.0, \"Max\": 9.5, \"FormatStr\": \"%.3f\" }, { \"ID\": \"afe0_p_3v3_G_min\", \"Num\": 83, \"Name\": \"afe0_p_3v3_G_min\", \"Desc\": \"\", \"Unit\": \"V\", \"Min\": 3.2, \"Max\": 3.4, \"FormatStr\": \"%.3f\" }, { \"ID\": \"afe0_p_3v3_G_avg\", \"Num\": 84, \"Name\": \"afe0_p_3v3_G_avg\", \"Desc\": \"\", \"Unit\": \"V\", \"Min\": 3.2, \"Max\": 3.4, \"FormatStr\": \"%.3f\" }, { \"ID\": \"afe0_p_3v3_G_max\", \"Num\": 85, \"Name\": \"afe0_p_3v3_G_max\", \"Desc\": \"\", \"Unit\": \"V\", \"Min\": 3.2, \"Max\": 3.4, \"FormatStr\": \"%.3f\" }, { \"ID\": \"afe0_p_v_protection_G_min\", \"Num\": 86, \"Name\": \"afe0_p_v_protection_G_min\", \"Desc\": \"\", \"Unit\": \"В\", \"Min\": 4.5, \"Max\": 5.5, \"FormatStr\": \"%.3f\" }, { \"ID\": \"afe0_p_v_protection_G_avg\", \"Num\": 87, \"Name\": \"afe0_p_v_protection_G_avg\", \"Desc\": \"\", \"Unit\": \"В\", \"Min\": 4.5, \"Max\": 5.5, \"FormatStr\": \"%.3f\" }, { \"ID\": \"afe0_p_v_protection_G_max\", \"Num\": 88, \"Name\": \"afe0_p_v_protection_G_max\", \"Desc\": \"\", \"Unit\": \"В\", \"Min\": 4.5, \"Max\": 5.5, \"FormatStr\": \"%.3f\" }, { \"ID\": \"afe0_m_v_protection_G_min\", \"Num\": 89, \"Name\": \"afe0_m_v_protection_G_min\", \"Desc\": \"\", \"Unit\": \"В\", \"Min\": -5.5, \"Max\": -4.5, \"FormatStr\": \"%.3f\" }, { \"ID\": \"afe0_m_v_protection_G_avg\", \"Num\": 90, \"Name\": \"afe0_m_v_protection_G_avg\", \"Desc\": \"\", \"Unit\": \"В\", \"Min\": -5.5, \"Max\": -4.5, \"FormatStr\": \"%.3f\" }, { \"ID\": \"afe0_m_v_protection_G_max\", \"Num\": 91, \"Name\": \"afe0_m_v_protection_G_max\", \"Desc\": \"\", \"Unit\": \"В\", \"Min\": -5.5, \"Max\": -4.5, \"FormatStr\": \"%.3f\" }, { \"ID\": \"afe0_p_5va_G_min\", \"Num\": 92, \"Name\": \"afe0_p_5va_G_min\", \"Desc\": \"\", \"Unit\": \"V\", \"Min\": 4.9, \"Max\": 5.1, \"FormatStr\": \"%.3f\" }, { \"ID\": \"afe0_p_5va_G_avg\", \"Num\": 93, \"Name\": \"afe0_p_5va_G_avg\", \"Desc\": \"\", \"Unit\": \"V\", \"Min\": 4.9, \"Max\": 5.1, \"FormatStr\": \"%.3f\" }, { \"ID\": \"afe0_p_5va_G_max\", \"Num\": 94, \"Name\": \"afe0_p_5va_G_max\", \"Desc\": \"\", \"Unit\": \"V\", \"Min\": 4.9, \"Max\": 5.1, \"FormatStr\": \"%.3f\" }, { \"ID\": \"afe0_m_5va_G_min\", \"Num\": 95, \"Name\": \"afe0_m_5va_G_min\", \"Desc\": \"\", \"Unit\": \"V\", \"Min\": -5.1, \"Max\": -4.9, \"FormatStr\": \"%.3f\" }, { \"ID\": \"afe0_m_5va_G_avg\", \"Num\": 96, \"Name\": \"afe0_m_5va_G_avg\", \"Desc\": \"\", \"Unit\": \"V\", \"Min\": -5.1, \"Max\": -4.9, \"FormatStr\": \"%.3f\" }, { \"ID\": \"afe0_m_5va_G_max\", \"Num\": 97, \"Name\": \"afe0_m_5va_G_max\", \"Desc\": \"\", \"Unit\": \"V\", \"Min\": -5.1, \"Max\": -4.9, \"FormatStr\": \"%.3f\" }, { \"ID\": \"afe1_p_20v_G_min\", \"Num\": 98, \"Name\": \"afe1_p_20v_G_min\", \"Desc\": \"\", \"Unit\": \"V\", \"Min\": 17.0, \"Max\": 19.0, \"FormatStr\": \"%.3f\" }, { \"ID\": \"afe1_p_20v_G_avg\", \"Num\": 99, \"Name\": \"afe1_p_20v_G_avg\", \"Desc\": \"\", \"Unit\": \"V\", \"Min\": 17.0, \"Max\": 19.0, \"FormatStr\": \"%.3f\" }, { \"ID\": \"afe1_p_20v_G_max\", \"Num\": 100, \"Name\": \"afe1_p_20v_G_max\", \"Desc\": \"\", \"Unit\": \"V\", \"Min\": 17.0, \"Max\": 19.0, \"FormatStr\": \"%.3f\" }, { \"ID\": \"afe1_p_8v_G_min\", \"Num\": 101, \"Name\": \"afe1_p_8v_G_min\", \"Desc\": \"\", \"Unit\": \"V\", \"Min\": 7.0, \"Max\": 9.5, \"FormatStr\": \"%.3f\" }, { \"ID\": \"afe1_p_8v_G_avg\", \"Num\": 102, \"Name\": \"afe1_p_8v_G_avg\", \"Desc\": \"\", \"Unit\": \"V\", \"Min\": 7.0, \"Max\": 9.5, \"FormatStr\": \"%.3f\" }, { \"ID\": \"afe1_p_8v_G_max\", \"Num\": 103, \"Name\": \"afe1_p_8v_G_max\", \"Desc\": \"\", \"Unit\": \"V\", \"Min\": 7.0, \"Max\": 9.5, \"FormatStr\": \"%.3f\" }, { \"ID\": \"afe1_p_3v3_G_min\", \"Num\": 104, \"Name\": \"afe1_p_3v3_G_min\", \"Desc\": \"\", \"Unit\": \"V\", \"Min\": 3.2, \"Max\": 3.4, \"FormatStr\": \"%.3f\" }, { \"ID\": \"afe1_p_3v3_G_avg\", \"Num\": 105, \"Name\": \"afe1_p_3v3_G_avg\", \"Desc\": \"\", \"Unit\": \"V\", \"Min\": 3.2, \"Max\": 3.4, \"FormatStr\": \"%.3f\" }, { \"ID\": \"afe1_p_3v3_G_max\", \"Num\": 106, \"Name\": \"afe1_p_3v3_G_max\", \"Desc\": \"\", \"Unit\": \"V\", \"Min\": 3.2, \"Max\": 3.4, \"FormatStr\": \"%.3f\" }, { \"ID\": \"afe1_p_v_protection_G_min\", \"Num\": 107, \"Name\": \"afe1_p_v_protection_G_min\", \"Desc\": \"\", \"Unit\": \"В\", \"Min\": 4.5, \"Max\": 5.5, \"FormatStr\": \"%.3f\" }, { \"ID\": \"afe1_p_v_protection_G_avg\", \"Num\": 108, \"Name\": \"afe1_p_v_protection_G_avg\", \"Desc\": \"\", \"Unit\": \"В\", \"Min\": 4.5, \"Max\": 5.5, \"FormatStr\": \"%.3f\" }, { \"ID\": \"afe1_p_v_protection_G_max\", \"Num\": 109, \"Name\": \"afe1_p_v_protection_G_max\", \"Desc\": \"\", \"Unit\": \"В\", \"Min\": 4.5, \"Max\": 5.5, \"FormatStr\": \"%.3f\" }, { \"ID\": \"afe1_m_v_protection_G_min\", \"Num\": 110, \"Name\": \"afe1_m_v_protection_G_min\", \"Desc\": \"\", \"Unit\": \"В\", \"Min\": -5.5, \"Max\": -4.5, \"FormatStr\": \"%.3f\" }, { \"ID\": \"afe1_m_v_protection_G_avg\", \"Num\": 111, \"Name\": \"afe1_m_v_protection_G_avg\", \"Desc\": \"\", \"Unit\": \"В\", \"Min\": -5.5, \"Max\": -4.5, \"FormatStr\": \"%.3f\" }, { \"ID\": \"afe1_m_v_protection_G_max\", \"Num\": 112, \"Name\": \"afe1_m_v_protection_G_max\", \"Desc\": \"\", \"Unit\": \"В\", \"Min\": -5.5, \"Max\": -4.5, \"FormatStr\": \"%.3f\" }, { \"ID\": \"afe1_p_5va_G_min\", \"Num\": 113, \"Name\": \"afe1_p_5va_G_min\", \"Desc\": \"\", \"Unit\": \"V\", \"Min\": 4.9, \"Max\": 5.1, \"FormatStr\": \"%.3f\" }, { \"ID\": \"afe1_p_5va_G_avg\", \"Num\": 114, \"Name\": \"afe1_p_5va_G_avg\", \"Desc\": \"\", \"Unit\": \"V\", \"Min\": 4.9, \"Max\": 5.1, \"FormatStr\": \"%.3f\" }, { \"ID\": \"afe1_p_5va_G_max\", \"Num\": 115, \"Name\": \"afe1_p_5va_G_max\", \"Desc\": \"\", \"Unit\": \"V\", \"Min\": 4.9, \"Max\": 5.1, \"FormatStr\": \"%.3f\" }, { \"ID\": \"afe1_m_5va_G_min\", \"Num\": 116, \"Name\": \"afe1_m_5va_G_min\", \"Desc\": \"\", \"Unit\": \"V\", \"Min\": -5.1, \"Max\": -4.9, \"FormatStr\": \"%.3f\" }, { \"ID\": \"afe1_m_5va_G_avg\", \"Num\": 117, \"Name\": \"afe1_m_5va_G_avg\", \"Desc\": \"\", \"Unit\": \"V\", \"Min\": -5.1, \"Max\": -4.9, \"FormatStr\": \"%.3f\" }, { \"ID\": \"afe1_m_5va_G_max\", \"Num\": 118, \"Name\": \"afe1_m_5va_G_max\", \"Desc\": \"\", \"Unit\": \"V\", \"Min\": -5.1, \"Max\": -4.9, \"FormatStr\": \"%.3f\" }, { \"ID\": \"pab0_m_12v_G_min\", \"Num\": 119, \"Name\": \"pab0_m_12v_G_min\", \"Desc\": \"\", \"Unit\": \"V\", \"Min\": -12.8, \"Max\": -11.2, \"FormatStr\": \"%.3f\" }, { \"ID\": \"pab0_m_12v_G_avg\", \"Num\": 120, \"Name\": \"pab0_m_12v_G_avg\", \"Desc\": \"\", \"Unit\": \"V\", \"Min\": -12.8, \"Max\": -11.2, \"FormatStr\": \"%.3f\" }, { \"ID\": \"pab0_m_12v_G_max\", \"Num\": 121, \"Name\": \"pab0_m_12v_G_max\", \"Desc\": \"\", \"Unit\": \"V\", \"Min\": -12.8, \"Max\": -11.2, \"FormatStr\": \"%.3f\" }, { \"ID\": \"pab0_m_20v_G_min\", \"Num\": 122, \"Name\": \"pab0_m_20v_G_min\", \"Desc\": \"\", \"Unit\": \"V\", \"Min\": -20.0, \"Max\": -17.0, \"FormatStr\": \"%.3f\" }, { \"ID\": \"pab0_m_20v_G_avg\", \"Num\": 123, \"Name\": \"pab0_m_20v_G_avg\", \"Desc\": \"\", \"Unit\": \"V\", \"Min\": -20.0, \"Max\": -17.0, \"FormatStr\": \"%.3f\" }, { \"ID\": \"pab0_m_20v_G_max\", \"Num\": 124, \"Name\": \"pab0_m_20v_G_max\", \"Desc\": \"\", \"Unit\": \"V\", \"Min\": -20.0, \"Max\": -17.0, \"FormatStr\": \"%.3f\" }, { \"ID\": \"pab0_p_5v_G_min\", \"Num\": 125, \"Name\": \"pab0_p_5v_G_min\", \"Desc\": \"\", \"Unit\": \"V\", \"Min\": 4.9, \"Max\": 5.1, \"FormatStr\": \"%.3f\" }, { \"ID\": \"pab0_p_5v_G_avg\", \"Num\": 126, \"Name\": \"pab0_p_5v_G_avg\", \"Desc\": \"\", \"Unit\": \"V\", \"Min\": 4.9, \"Max\": 5.1, \"FormatStr\": \"%.3f\" }, { \"ID\": \"pab0_p_5v_G_max\", \"Num\": 127, \"Name\": \"pab0_p_5v_G_max\", \"Desc\": \"\", \"Unit\": \"V\", \"Min\": 4.9, \"Max\": 5.1, \"FormatStr\": \"%.3f\" }, { \"ID\": \"pab0_p_8v_G_min\", \"Num\": 128, \"Name\": \"pab0_p_8v_G_min\", \"Desc\": \"\", \"Unit\": \"V\", \"Min\": 7.0, \"Max\": 9.5, \"FormatStr\": \"%.3f\" }, { \"ID\": \"pab0_p_8v_G_avg\", \"Num\": 129, \"Name\": \"pab0_p_8v_G_avg\", \"Desc\": \"\", \"Unit\": \"V\", \"Min\": 7.0, \"Max\": 9.5, \"FormatStr\": \"%.3f\" }, { \"ID\": \"pab0_p_8v_G_max\", \"Num\": 130, \"Name\": \"pab0_p_8v_G_max\", \"Desc\": \"\", \"Unit\": \"V\", \"Min\": 7.0, \"Max\": 9.5, \"FormatStr\": \"%.3f\" }, { \"ID\": \"pab0_p_15v_G_min\", \"Num\": 131, \"Name\": \"pab0_p_15v_G_min\", \"Desc\": \"\", \"Unit\": \"V\", \"Min\": 15.5, \"Max\": 14.5, \"FormatStr\": \"%.3f\" }, { \"ID\": \"pab0_p_15v_G_avg\", \"Num\": 132, \"Name\": \"pab0_p_15v_G_avg\", \"Desc\": \"\", \"Unit\": \"V\", \"Min\": 15.5, \"Max\": 14.5, \"FormatStr\": \"%.3f\" }, { \"ID\": \"pab0_p_15v_G_max\", \"Num\": 133, \"Name\": \"pab0_p_15v_G_max\", \"Desc\": \"\", \"Unit\": \"V\", \"Min\": 15.5, \"Max\": 14.5, \"FormatStr\": \"%.3f\" }, { \"ID\": \"pab0_p_20v_G_min\", \"Num\": 134, \"Name\": \"pab0_p_20v_G_min\", \"Desc\": \"\", \"Unit\": \"V\", \"Min\": 17.0, \"Max\": 19.0, \"FormatStr\": \"%.3f\" }, { \"ID\": \"pab0_p_20v_G_avg\", \"Num\": 135, \"Name\": \"pab0_p_20v_G_avg\", \"Desc\": \"\", \"Unit\": \"V\", \"Min\": 17.0, \"Max\": 19.0, \"FormatStr\": \"%.3f\" }, { \"ID\": \"pab0_p_20v_G_max\", \"Num\": 136, \"Name\": \"pab0_p_20v_G_max\", \"Desc\": \"\", \"Unit\": \"V\", \"Min\": 17.0, \"Max\": 19.0, \"FormatStr\": \"%.3f\" }, { \"ID\": \"pab0_p_hv_G_min\", \"Num\": 137, \"Name\": \"pab0_p_hv_G_min\", \"Desc\": \"\", \"Unit\": \"V\", \"Min\": 15.0, \"Max\": 205.0, \"FormatStr\": \"%.1f\" }, { \"ID\": \"pab0_p_hv_G_avg\", \"Num\": 138, \"Name\": \"pab0_p_hv_G_avg\", \"Desc\": \"\", \"Unit\": \"V\", \"Min\": 15.0, \"Max\": 205.0, \"FormatStr\": \"%.1f\" }, { \"ID\": \"pab0_p_hv_G_max\", \"Num\": 139, \"Name\": \"pab0_p_hv_G_max\", \"Desc\": \"\", \"Unit\": \"V\", \"Min\": 15.0, \"Max\": 205.0, \"FormatStr\": \"%.1f\" }, { \"ID\": \"pab0_p_220v_G_min\", \"Num\": 140, \"Name\": \"pab0_p_220v_G_min\", \"Desc\": \"\", \"Unit\": \"V\", \"Min\": 215.0, \"Max\": 230.0, \"FormatStr\": \"%.3f\" }, { \"ID\": \"pab0_p_220v_G_avg\", \"Num\": 141, \"Name\": \"pab0_p_220v_G_avg\", \"Desc\": \"\", \"Unit\": \"V\", \"Min\": 215.0, \"Max\": 230.0, \"FormatStr\": \"%.3f\" }, { \"ID\": \"pab0_p_220v_G_max\", \"Num\": 142, \"Name\": \"pab0_p_220v_G_max\", \"Desc\": \"\", \"Unit\": \"V\", \"Min\": 215.0, \"Max\": 230.0, \"FormatStr\": \"%.3f\" }, { \"ID\": \"pab1_m_12v_G_min\", \"Num\": 143, \"Name\": \"pab1_m_12v_G_min\", \"Desc\": \"\", \"Unit\": \"V\", \"Min\": -12.8, \"Max\": -11.2, \"FormatStr\": \"%.3f\" }, { \"ID\": \"pab1_m_12v_G_avg\", \"Num\": 144, \"Name\": \"pab1_m_12v_G_avg\", \"Desc\": \"\", \"Unit\": \"V\", \"Min\": -12.8, \"Max\": -11.2, \"FormatStr\": \"%.3f\" }, { \"ID\": \"pab1_m_12v_G_max\", \"Num\": 145, \"Name\": \"pab1_m_12v_G_max\", \"Desc\": \"\", \"Unit\": \"V\", \"Min\": -12.8, \"Max\": -11.2, \"FormatStr\": \"%.3f\" }, { \"ID\": \"pab1_m_20v_G_min\", \"Num\": 146, \"Name\": \"pab1_m_20v_G_min\", \"Desc\": \"\", \"Unit\": \"V\", \"Min\": -20.0, \"Max\": -17.0, \"FormatStr\": \"%.3f\" }, { \"ID\": \"pab1_m_20v_G_avg\", \"Num\": 147, \"Name\": \"pab1_m_20v_G_avg\", \"Desc\": \"\", \"Unit\": \"V\", \"Min\": -20.0, \"Max\": -17.0, \"FormatStr\": \"%.3f\" }, { \"ID\": \"pab1_m_20v_G_max\", \"Num\": 148, \"Name\": \"pab1_m_20v_G_max\", \"Desc\": \"\", \"Unit\": \"V\", \"Min\": -20.0, \"Max\": -17.0, \"FormatStr\": \"%.3f\" }, { \"ID\": \"pab1_p_5v_G_min\", \"Num\": 149, \"Name\": \"pab1_p_5v_G_min\", \"Desc\": \"\", \"Unit\": \"V\", \"Min\": 4.9, \"Max\": 5.1, \"FormatStr\": \"%.3f\" }, { \"ID\": \"pab1_p_5v_G_avg\", \"Num\": 150, \"Name\": \"pab1_p_5v_G_avg\", \"Desc\": \"\", \"Unit\": \"V\", \"Min\": 4.9, \"Max\": 5.1, \"FormatStr\": \"%.3f\" }, { \"ID\": \"pab1_p_5v_G_max\", \"Num\": 151, \"Name\": \"pab1_p_5v_G_max\", \"Desc\": \"\", \"Unit\": \"V\", \"Min\": 4.9, \"Max\": 5.1, \"FormatStr\": \"%.3f\" }, { \"ID\": \"pab1_p_8v_G_min\", \"Num\": 152, \"Name\": \"pab1_p_8v_G_min\", \"Desc\": \"\", \"Unit\": \"V\", \"Min\": 7.0, \"Max\": 9.5, \"FormatStr\": \"%.3f\" }, { \"ID\": \"pab1_p_8v_G_avg\", \"Num\": 153, \"Name\": \"pab1_p_8v_G_avg\", \"Desc\": \"\", \"Unit\": \"V\", \"Min\": 7.0, \"Max\": 9.5, \"FormatStr\": \"%.3f\" }, { \"ID\": \"pab1_p_8v_G_max\", \"Num\": 154, \"Name\": \"pab1_p_8v_G_max\", \"Desc\": \"\", \"Unit\": \"V\", \"Min\": 7.0, \"Max\": 9.5, \"FormatStr\": \"%.3f\" }, { \"ID\": \"pab1_p_15v_G_min\", \"Num\": 155, \"Name\": \"pab1_p_15v_G_min\", \"Desc\": \"\", \"Unit\": \"V\", \"Min\": 15.5, \"Max\": 14.5, \"FormatStr\": \"%.3f\" }, { \"ID\": \"pab1_p_15v_G_avg\", \"Num\": 156, \"Name\": \"pab1_p_15v_G_avg\", \"Desc\": \"\", \"Unit\": \"V\", \"Min\": 15.5, \"Max\": 14.5, \"FormatStr\": \"%.3f\" }, { \"ID\": \"pab1_p_15v_G_max\", \"Num\": 157, \"Name\": \"pab1_p_15v_G_max\", \"Desc\": \"\", \"Unit\": \"V\", \"Min\": 15.5, \"Max\": 14.5, \"FormatStr\": \"%.3f\" }, { \"ID\": \"pab1_p_20v_G_min\", \"Num\": 158, \"Name\": \"pab1_p_20v_G_min\", \"Desc\": \"\", \"Unit\": \"V\", \"Min\": 17.0, \"Max\": 19.0, \"FormatStr\": \"%.3f\" }, { \"ID\": \"pab1_p_20v_G_avg\", \"Num\": 159, \"Name\": \"pab1_p_20v_G_avg\", \"Desc\": \"\", \"Unit\": \"V\", \"Min\": 17.0, \"Max\": 19.0, \"FormatStr\": \"%.3f\" }, { \"ID\": \"pab1_p_20v_G_max\", \"Num\": 160, \"Name\": \"pab1_p_20v_G_max\", \"Desc\": \"\", \"Unit\": \"V\", \"Min\": 17.0, \"Max\": 19.0, \"FormatStr\": \"%.3f\" }, { \"ID\": \"pab1_p_hv_G_min\", \"Num\": 161, \"Name\": \"pab1_p_hv_G_min\", \"Desc\": \"\", \"Unit\": \"V\", \"Min\": 15.0, \"Max\": 205.0, \"FormatStr\": \"%.1f\" }, { \"ID\": \"pab1_p_hv_G_avg\", \"Num\": 162, \"Name\": \"pab1_p_hv_G_avg\", \"Desc\": \"\", \"Unit\": \"V\", \"Min\": 15.0, \"Max\": 205.0, \"FormatStr\": \"%.1f\" }, { \"ID\": \"pab1_p_hv_G_max\", \"Num\": 163, \"Name\": \"pab1_p_hv_G_max\", \"Desc\": \"\", \"Unit\": \"V\", \"Min\": 15.0, \"Max\": 205.0, \"FormatStr\": \"%.1f\" }, { \"ID\": \"pab1_p_220v_G_min\", \"Num\": 164, \"Name\": \"pab1_p_220v_G_min\", \"Desc\": \"\", \"Unit\": \"V\", \"Min\": 215.0, \"Max\": 230.0, \"FormatStr\": \"%.3f\" }, { \"ID\": \"pab1_p_220v_G_avg\", \"Num\": 165, \"Name\": \"pab1_p_220v_G_avg\", \"Desc\": \"\", \"Unit\": \"V\", \"Min\": 215.0, \"Max\": 230.0, \"FormatStr\": \"%.3f\" }, { \"ID\": \"pab1_p_220v_G_max\", \"Num\": 166, \"Name\": \"pab1_p_220v_G_max\", \"Desc\": \"\", \"Unit\": \"V\", \"Min\": 215.0, \"Max\": 230.0, \"FormatStr\": \"%.3f\" }, { \"ID\": \"TelPMD2Up_time\", \"Num\": 167, \"Name\": \"PM D2 Uptime\", \"Desc\": \"\", \"Unit\": \"\", \"FormatStr\": \"%t\" }, { \"ID\": \"TelPMD6Up_time\", \"Num\": 168, \"Name\": \"PM D6 Uptime\", \"Desc\": \"\", \"Unit\": \"\", \"FormatStr\": \"%t\" }, { \"ID\": \"rb0_time\", \"Num\": 169, \"Name\": \"rb0 Uptime\", \"Desc\": \"\", \"Unit\": \"\", \"FormatStr\": \"%t\" }, { \"ID\": \"rb1_time\", \"Num\": 170, \"Name\": \"rb1 Uptime\", \"Desc\": \"\", \"Unit\": \"\", \"FormatStr\": \"%t\" }, { \"ID\": \"afe0_time\", \"Num\": 171, \"Name\": \"afe0 Uptime\", \"Desc\": \"\", \"Unit\": \"\", \"FormatStr\": \"%t\" }, { \"ID\": \"afe1_time\", \"Num\": 172, \"Name\": \"afe1 Uptime\", \"Desc\": \"\", \"Unit\": \"\", \"FormatStr\": \"%t\" }, { \"ID\": \"pab0_time\", \"Num\": 173, \"Name\": \"pab0 Uptime\", \"Desc\": \"\", \"Unit\": \"\", \"FormatStr\": \"%t\" }, { \"ID\": \"pab1_time\", \"Num\": 174, \"Name\": \"pab1 Uptime\", \"Desc\": \"\", \"Unit\": \"\", \"FormatStr\": \"%t\" }, { \"ID\": \"TelPMPassPacketCount\", \"Num\": 175, \"Name\": \"TelPMPassPacketCount\", \"Desc\": \"\", \"Unit\": \"\", \"FormatStr\": \"%.0f\" }, { \"ID\": \"TelRB0PassPacketCount\", \"Num\": 176, \"Name\": \"TelRB0PassPacketCount\", \"Desc\": \"\", \"Unit\": \"\", \"FormatStr\": \"%.0f\" }, { \"ID\": \"TelRB1PassPacketCount\", \"Num\": 177, \"Name\": \"TelRB1PassPacketCount\", \"Desc\": \"\", \"Unit\": \"\", \"FormatStr\": \"%.0f\" }, { \"ID\": \"TelAFE0PassPacketCount\", \"Num\": 178, \"Name\": \"TelAFE0PassPacketCount\", \"Desc\": \"\", \"Unit\": \"\", \"FormatStr\": \"%.0f\" }, { \"ID\": \"TelAFE1PassPacketCount\", \"Num\": 179, \"Name\": \"TelAFE1PassPacketCount\", \"Desc\": \"\", \"Unit\": \"\", \"FormatStr\": \"%.0f\" }, { \"ID\": \"TelPAB0PassPacketCount\", \"Num\": 180, \"Name\": \"TelPAB0PassPacketCount\", \"Desc\": \"\", \"Unit\": \"\", \"FormatStr\": \"%.0f\" }, { \"ID\": \"TelPAB1PassPacketCount\", \"Num\": 181, \"Name\": \"TelPAB1PassPacketCount\", \"Desc\": \"\", \"Unit\": \"\", \"FormatStr\": \"%.0f\" }, { \"ID\": \"TelPMErrorPacketCount\", \"Num\": 182, \"Name\": \"TelPMErrorPacketCount\", \"Desc\": \"\", \"Unit\": \"\", \"FormatStr\": \"%.0f\" }, { \"ID\": \"TelRB0ErrorPacketCount\", \"Num\": 183, \"Name\": \"TelRB0ErrorPacketCount\", \"Desc\": \"\", \"Unit\": \"\", \"FormatStr\": \"%.0f\" }, { \"ID\": \"TelRB1ErrorPacketCount\", \"Num\": 184, \"Name\": \"TelRB1ErrorPacketCount\", \"Desc\": \"\", \"Unit\": \"\", \"FormatStr\": \"%.0f\" }, { \"ID\": \"TelAFE0ErrorPacketCount\", \"Num\": 185, \"Name\": \"TelAFE0ErrorPacketCount\", \"Desc\": \"\", \"Unit\": \"\", \"FormatStr\": \"%.0f\" }, { \"ID\": \"TelAFE1ErrorPacketCount\", \"Num\": 186, \"Name\": \"TelAFE1ErrorPacketCount\", \"Desc\": \"\", \"Unit\": \"\", \"FormatStr\": \"%.0f\" }, { \"ID\": \"TelPAB0ErrorPacketCount\", \"Num\": 187, \"Name\": \"TelPAB0ErrorPacketCount\", \"Desc\": \"\", \"Unit\": \"\", \"FormatStr\": \"%.0f\" }, { \"ID\": \"TelPAB1ErrorPacketCount\", \"Num\": 188, \"Name\": \"TelPAB1ErrorPacketCount\", \"Desc\": \"\", \"Unit\": \"\", \"FormatStr\": \"%.0f\" }, { \"ID\": \"_FrameFormatVersion\", \"Num\": 189, \"Name\": \"Frame Format Version\", \"Desc\": \"Версия формата пакета\", \"Unit\": \"\", \"FormatStr\": \"%.0f\" }, { \"ID\": \"_Ncycle\", \"Num\": 190, \"Name\": \"N cycle\", \"Desc\": \"Номер цикла\", \"Unit\": \"\", \"FormatStr\": \"%.0f\" }, { \"ID\": \"_Ntick\", \"Num\": 191, \"Name\": \"N tick\", \"Desc\": \"Номер такта в цикле\", \"Unit\": \"\", \"FormatStr\": \"%.0f\" }, { \"ID\": \"_GlobalTime1\", \"Num\": 192, \"Name\": \"Global Time 1\", \"Type\": \"DateTime\", \"Desc\": \"Метка времени, количество секунд с момента начала эпохи Unix\", \"Unit\": \"Unix time\", \"FormatStr\": \"%.0f\" }, { \"ID\": \"_GlobalTime2\", \"Num\": 193, \"Name\": \"Global Time 2\", \"Desc\": \"Метка времени, количество наносекунд с момента начала текущей секунды\", \"Unit\": \"\", \"FormatStr\": \"%.0f\" }, { \"ID\": \"_Nchanel\", \"Num\": 194, \"Name\": \"N chanel\", \"Desc\": \"Номер канала (приемника)\", \"Unit\": \"\", \"FormatStr\": \"%.0f\" }, { \"ID\": \"_ScanDurationP\", \"Num\": 195, \"Name\": \"Scan Duration\", \"Desc\": \"Длительность области сканирования (в парах семплов)\", \"Unit\": \"пар семплов\", \"FormatStr\": \"%.0f\" }, { \"ID\": \"_CRC8\", \"Num\": 196, \"Name\": \"CRC8\", \"Desc\": \"Контрольная сумма CRC-8-CCITT 8-бит\", \"Unit\": \"\", \"FormatStr\": \"%.0f\" }, { \"ID\": \"_CRC8_calculated\", \"Num\": 197, \"Name\": \"CRC8 расчетный\", \"Desc\": \"Счетчик сформированных пакетов\", \"Unit\": \"\", \"FormatStr\": \"%.0f\" }, { \"ID\": \"_ScanDelayP\", \"Num\": 198, \"Name\": \"Scan Delay\", \"Desc\": \"Задержка области сканирования\", \"Unit\": \"отчет\", \"FormatStr\": \"%.0f\" }, { \"ID\": \"_MuxRX\", \"Num\": 199, \"Name\": \"Mux RX\", \"Desc\": \"Состояние мультиплексора приемника\", \"Unit\": \"\", \"FormatStr\": \"%.0f\" }, { \"ID\": \"_MuxTX\", \"Num\": 200, \"Name\": \"Mux TX\", \"Desc\": \"Cостояние мультиплексора передатчика\", \"Unit\": \"\", \"FormatStr\": \"%.0f\" }, { \"ID\": \"_EncodersParam1\", \"Num\": 201, \"Name\": \"Encoders Param 1\", \"Desc\": \"Состояние энкодера входа синхронизации №1\", \"Unit\": \"\", \"FormatStr\": \"%.0f\" }, { \"ID\": \"_EncodersParam2\", \"Num\": 202, \"Name\": \"Encoders Param 2\", \"Desc\": \"Состояние энкодера входа синхронизации №2\", \"Unit\": \"\", \"FormatStr\": \"%.0f\" }, { \"ID\": \"_LosePacket\", \"Num\": 203, \"Name\": \"Lose Packet\", \"Desc\": \"Количество пропущенных А-сканов\", \"Unit\": \"\", \"FormatStr\": \"%.0f\" }, { \"ID\": \"_SampleInterval\", \"Num\": 204, \"Name\": \"Sample Interval\", \"Desc\": \"Интервал следования семплов\", \"Unit\": \"с\", \"FormatStr\": \"%g\" }, { \"ID\": \"_GainCoeff\", \"Num\": 205, \"Name\": \"Gain Coeff\", \"Desc\": \"Коэффициент усиления предварительных усилителей\", \"Unit\": \"дБ\", \"FormatStr\": \"%.2f\" }, { \"ID\": \"_PacketCounter\", \"Num\": 206, \"Name\": \"Packet Counter\", \"Desc\": \"Счетчик сформированных пакетов\", \"Unit\": \"\", \"FormatStr\": \"%.0f\" }, { \"ID\": \"_Encoder1CurrData_PL0\", \"Num\": 207, \"Name\": \"Encoder1CurrData_PL0\", \"Desc\": \"Текущее значение счетчика энкодера 1 ПЛИС 0\", \"Unit\": \"\", \"FormatStr\": \"%.0f\" }, { \"ID\": \"_Encoder1CurrData_PL1\", \"Num\": 208, \"Name\": \"Encoder1CurrData_PL1\", \"Desc\": \"Текущее значение счетчика энкодера 1 ПЛИС 1\", \"Unit\": \"\", \"FormatStr\": \"%.0f\" }, { \"ID\": \"_Encoder2CurrData_PL0\", \"Num\": 209, \"Name\": \"Encoder2CurrData_PL0\", \"Desc\": \"Текущее значение счетчика энкодера 2 ПЛИС 0\", \"Unit\": \"\", \"FormatStr\": \"%.0f\" }, { \"ID\": \"_Encoder2CurrData_PL1\", \"Num\": 210, \"Name\": \"Encoder2CurrData_PL1\", \"Desc\": \"Текущее значение счетчика энкодера 2 ПЛИС 1\", \"Unit\": \"\", \"FormatStr\": \"%.0f\" }, { \"ID\": \"_PulseCurrData_PL0\", \"Num\": 211, \"Name\": \"PulseCurrData_PL0\", \"Desc\": \"Текущее значение счетчика импульсов ПЛИС 0\", \"Unit\": \"\", \"FormatStr\": \"%.0f\" }, { \"ID\": \"_PulseCurrData_PL1\", \"Num\": 212, \"Name\": \"PulseCurrData_PL1\", \"Desc\": \"Текущее значение счетчика импульсов ПЛИС 1\", \"Unit\": \"\", \"FormatStr\": \"%.0f\" }, { \"ID\": \"_NumOfRuns_PL0\", \"Num\": 213, \"Name\": \"NumOfRuns_PL0\", \"Desc\": \"Текущее значение счетчика количества запусков цикла ПЛИС 0\", \"Unit\": \"\", \"FormatStr\": \"%.0f\" }, { \"ID\": \"_NumOfRuns_PL1\", \"Num\": 214, \"Name\": \"NumOfRuns_PL1\", \"Desc\": \"Текущее значение счетчика количества запусков цикла ПЛИС 1\", \"Unit\": \"\", \"FormatStr\": \"%.0f\" }, { \"ID\": \"_Encoder1ScalingFactor_PL0\", \"Num\": 215, \"Name\": \"Encoder1ScalingFactor_PL0\", \"Desc\": \"Encoder1ScalingFactor_PL0\", \"Unit\": \"\", \"FormatStr\": \"%.0f\" }, { \"ID\": \"_TelRAMTestCompletionPercentage\", \"Num\": 216, \"Name\": \"TelRAMTestCompletionPercentage\", \"Desc\": \"\", \"Unit\": \"\", \"FormatStr\": \"%.2f\" }, { \"ID\": \"_NumberOfApplicationLaunches\", \"Num\": 217, \"Name\": \"NumberOfApplicationLaunches\", \"Desc\": \"\", \"Unit\": \"\", \"FormatStr\": \"%.0f\" }, { \"ID\": \"_TotalOperatingTime\", \"Num\": 218, \"Name\": \"TotalOperatingTime [min]\", \"Desc\": \"\", \"Unit\": \"\", \"FormatStr\": \"%.0f\" }, { \"ID\": \"_NumberOfFileRecords\", \"Num\": 219, \"Name\": \"NumberOfFileRecords\", \"Desc\": \"\", \"Unit\": \"\", \"FormatStr\": \"%.0f\" } ], \"Table\": [ { \"Num\": 0, \"Access\": \"rw\", \"ColumnCount\": 32, \"NeedParamPrepare\": false, \"Columns\": [ { \"Column\": 0, \"Desc\": \"Такт №1 в цикле\", \"Name\": \"1\" }, { \"Column\": 1, \"Desc\": \"Такт №2 в цикле\", \"Name\": \"2\" }, { \"Column\": 2, \"Desc\": \"Такт №3 в цикле\", \"Name\": \"3\" }, { \"Column\": 3, \"Desc\": \"Такт №4 в цикле\", \"Name\": \"4\" }, { \"Column\": 4, \"Desc\": \"Такт №5 в цикле\", \"Name\": \"5\" }, { \"Column\": 5, \"Desc\": \"Такт №6 в цикле\", \"Name\": \"6\" }, { \"Column\": 6, \"Desc\": \"Такт №7 в цикле\", \"Name\": \"7\" }, { \"Column\": 7, \"Desc\": \"Такт №8 в цикле\", \"Name\": \"8\" }, { \"Column\": 8, \"Desc\": \"Такт №9 в цикле\", \"Name\": \"9\" }, { \"Column\": 9, \"Desc\": \"Такт №10 в цикле\", \"Name\": \"10\" }, { \"Column\": 10, \"Desc\": \"Такт №11 в цикле\", \"Name\": \"11\" }, { \"Column\": 11, \"Desc\": \"Такт №12 в цикле\", \"Name\": \"12\" }, { \"Column\": 12, \"Desc\": \"Такт №13 в цикле\", \"Name\": \"13\" }, { \"Column\": 13, \"Desc\": \"Такт №14 в цикле\", \"Name\": \"14\" }, { \"Column\": 14, \"Desc\": \"Такт №15 в цикле\", \"Name\": \"15\" }, { \"Column\": 15, \"Desc\": \"Такт №16 в цикле\", \"Name\": \"16\" }, { \"Column\": 16, \"Desc\": \"Такт №17 в цикле\", \"Name\": \"17\" }, { \"Column\": 17, \"Desc\": \"Такт №18 в цикле\", \"Name\": \"18\" }, { \"Column\": 18, \"Desc\": \"Такт №19 в цикле\", \"Name\": \"19\" }, { \"Column\": 19, \"Desc\": \"Такт №20 в цикле\", \"Name\": \"20\" }, { \"Column\": 20, \"Desc\": \"Такт №21 в цикле\", \"Name\": \"21\" }, { \"Column\": 21, \"Desc\": \"Такт №22 в цикле\", \"Name\": \"22\" }, { \"Column\": 22, \"Desc\": \"Такт №23 в цикле\", \"Name\": \"23\" }, { \"Column\": 23, \"Desc\": \"Такт №24 в цикле\", \"Name\": \"24\" }, { \"Column\": 24, \"Desc\": \"Такт №25 в цикле\", \"Name\": \"25\" }, { \"Column\": 25, \"Desc\": \"Такт №26 в цикле\", \"Name\": \"26\" }, { \"Column\": 26, \"Desc\": \"Такт №27 в цикле\", \"Name\": \"27\" }, { \"Column\": 27, \"Desc\": \"Такт №28 в цикле\", \"Name\": \"28\" }, { \"Column\": 28, \"Desc\": \"Такт №29 в цикле\", \"Name\": \"29\" }, { \"Column\": 29, \"Desc\": \"Такт №30 в цикле\", \"Name\": \"30\" }, { \"Column\": 30, \"Desc\": \"Такт №31 в цикле\", \"Name\": \"31\" }, { \"Column\": 31, \"Desc\": \"Такт №32 в цикле\", \"Name\": \"32\" } ], \"DataType\": \"float\", \"FormatStr\": \"%g\", \"ID\": \"CCTicksSet1F\", \"Name\": \"Параметры цикла для каналов от 1 до 8\", \"RowCount\": 10, \"Rows\": [ { \"Desc\": \"Разрешить формирование импульса возбуждения ПЭП № от 1 до 8\", \"ID\": \"Generator1Enable\", \"Max\": 1, \"Min\": 0, \"Name\": \"Разрешить работу ГИ №1\", \"Row\": 0, \"Unit\": \"\" }, { \"Desc\": \"Номер ПЭП (с 1 по 8) подключаемый к выходу генератора импульсов возбуждения № 1\", \"ID\": \"Generator1Multiplexer\", \"Max\": 8, \"Min\": 1, \"Name\": \"№ ПЭП (с 1 по 8) подключенный к ГИ №1\", \"Row\": 1, \"Unit\": \"\" }, { \"Desc\": \"Значение задержки импульса возбуждения ПЭП на выходе ГИ №1\", \"ID\": \"Generator1PulseDelay\", \"Max\": 30, \"Min\": 0, \"Name\": \"Задержка импульса ГИ №1\", \"Row\": 2, \"Unit\": \"мкс\" }, { \"Desc\": \"Значение длительности импульса возбуждения ПЭП на выходе ГИ №1\", \"ID\": \"Generator1PulseDuration\", \"Max\": 1, \"Min\": 0.05, \"Name\": \"Длительность импульса ГИ\", \"Row\": 3, \"Unit\": \"мкс\" }, { \"Desc\": \"Разрешение работы приемника №1 сигнала ПЭП, формирование А-скана и передачу пакета с данными на ПК\", \"ID\": \"Receiver1Enable\", \"Max\": 1, \"Min\": 0, \"Name\": \"Разрешить работу приемника\", \"Row\": 4, \"Unit\": \"\" }, { \"Desc\": \"Номер ПЭП (с 1 по 8) подключенный ко входу приемника № 1\", \"ID\": \"Receiver1Multiplexer\", \"Max\": 8, \"Min\": 1, \"Name\": \"№ ПЭП (с 1 по 8) подключенный к приемнику №1\", \"Row\": 5, \"Unit\": \"\" }, { \"Desc\": \"Задержка начала развертки сигнала приемника №1 в такте\", \"ID\": \"ScanDelay1\", \"Max\": 200, \"Min\": 0, \"Name\": \"Задержка развертки приемника №1\", \"Row\": 6, \"Unit\": \"мкс\" }, { \"Desc\": \"Длительность записи сигнала приемника №1 в такте\", \"ID\": \"ScanDuration1\", \"Max\": 80, \"Min\": 1, \"Name\": \"Длительность развертки приемника №1\", \"Row\": 7, \"Unit\": \"мкс\" }, { \"Desc\": \"Коэффициент усиления предварительного усилителя приемника сигналов ПЭП №1\", \"ID\": \"Receiver1StaticGain\", \"Max\": 100, \"Min\": -100, \"Name\": \"Коэффициент усиления приемника №1\", \"Row\": 8, \"Unit\": \"дБ\" }, { \"Desc\": \"Выходное значение ЦАП №1\", \"ID\": \"Receiver1StaticGain\", \"Max\": 1023, \"Min\": 0, \"Name\": \"Выходное значение ЦАП №1 управляющий коэффициентом усиления приемника №1\", \"Row\": 9, \"Unit\": \"отсчет\" } ], \"Type\": \"Float\" }, { \"Num\": 1, \"Access\": \"rw\", \"ColumnCount\": 32, \"NeedParamPrepare\": false, \"Columns\": [ { \"Column\": 0, \"Desc\": \"Такт №1 в цикле\", \"Name\": \"1\" }, { \"Column\": 1, \"Desc\": \"Такт №2 в цикле\", \"Name\": \"2\" }, { \"Column\": 2, \"Desc\": \"Такт №3 в цикле\", \"Name\": \"3\" }, { \"Column\": 3, \"Desc\": \"Такт №4 в цикле\", \"Name\": \"4\" }, { \"Column\": 4, \"Desc\": \"Такт №5 в цикле\", \"Name\": \"5\" }, { \"Column\": 5, \"Desc\": \"Такт №6 в цикле\", \"Name\": \"6\" }, { \"Column\": 6, \"Desc\": \"Такт №7 в цикле\", \"Name\": \"7\" }, { \"Column\": 7, \"Desc\": \"Такт №8 в цикле\", \"Name\": \"8\" }, { \"Column\": 8, \"Desc\": \"Такт №9 в цикле\", \"Name\": \"9\" }, { \"Column\": 9, \"Desc\": \"Такт №10 в цикле\", \"Name\": \"10\" }, { \"Column\": 10, \"Desc\": \"Такт №11 в цикле\", \"Name\": \"11\" }, { \"Column\": 11, \"Desc\": \"Такт №12 в цикле\", \"Name\": \"12\" }, { \"Column\": 12, \"Desc\": \"Такт №13 в цикле\", \"Name\": \"13\" }, { \"Column\": 13, \"Desc\": \"Такт №14 в цикле\", \"Name\": \"14\" }, { \"Column\": 14, \"Desc\": \"Такт №15 в цикле\", \"Name\": \"15\" }, { \"Column\": 15, \"Desc\": \"Такт №16 в цикле\", \"Name\": \"16\" }, { \"Column\": 16, \"Desc\": \"Такт №17 в цикле\", \"Name\": \"17\" }, { \"Column\": 17, \"Desc\": \"Такт №18 в цикле\", \"Name\": \"18\" }, { \"Column\": 18, \"Desc\": \"Такт №19 в цикле\", \"Name\": \"19\" }, { \"Column\": 19, \"Desc\": \"Такт №20 в цикле\", \"Name\": \"20\" }, { \"Column\": 20, \"Desc\": \"Такт №21 в цикле\", \"Name\": \"21\" }, { \"Column\": 21, \"Desc\": \"Такт №22 в цикле\", \"Name\": \"22\" }, { \"Column\": 22, \"Desc\": \"Такт №23 в цикле\", \"Name\": \"23\" }, { \"Column\": 23, \"Desc\": \"Такт №24 в цикле\", \"Name\": \"24\" }, { \"Column\": 24, \"Desc\": \"Такт №25 в цикле\", \"Name\": \"25\" }, { \"Column\": 25, \"Desc\": \"Такт №26 в цикле\", \"Name\": \"26\" }, { \"Column\": 26, \"Desc\": \"Такт №27 в цикле\", \"Name\": \"27\" }, { \"Column\": 27, \"Desc\": \"Такт №28 в цикле\", \"Name\": \"28\" }, { \"Column\": 28, \"Desc\": \"Такт №29 в цикле\", \"Name\": \"29\" }, { \"Column\": 29, \"Desc\": \"Такт №30 в цикле\", \"Name\": \"30\" }, { \"Column\": 30, \"Desc\": \"Такт №31 в цикле\", \"Name\": \"31\" }, { \"Column\": 31, \"Desc\": \"Такт №32 в цикле\", \"Name\": \"32\" } ], \"DataType\": \"float\", \"FormatStr\": \"%g\", \"ID\": \"CCTicksSet2F\", \"Name\": \"Параметры цикла для каналов от 9 до 16\", \"RowCount\": 10, \"Rows\": [ { \"Desc\": \"Разрешить формирование импульса возбуждения для ПЭП № от 9 до 16\", \"ID\": \"Generator2Enable\", \"Max\": 1, \"Min\": 0, \"Name\": \"Разрешить работу ГИ №2\", \"Row\": 0, \"Unit\": \"\" }, { \"Desc\": \"Номер ПЭП (с 9 по 16) подключаемый к выходу генератора импульсов возбуждения № 2\", \"ID\": \"Generator2Multiplexer\", \"Max\": 16, \"Min\": 9, \"Name\": \"№ ПЭП (с 9 по 16) подключенный к ГИ №2\", \"Row\": 1, \"Unit\": \"\" }, { \"Desc\": \"Значение задержки импульса возбуждения ПЭП на выходе ГИ №2\", \"ID\": \"Generator2PulseDelay\", \"Max\": 30, \"Min\": 0, \"Name\": \"Задержка импульса ГИ №2\", \"Row\": 2, \"Unit\": \"мкс\" }, { \"Desc\": \"Значение длительности импульса возбуждения ПЭП на выходе ГИ №2\", \"ID\": \"Generator2PulseDuration\", \"Max\": 1, \"Min\": 0.05, \"Name\": \"Длительность импульса ГИ\", \"Row\": 3, \"Unit\": \"мкс\" }, { \"Desc\": \"Разрешение работы приемника №2 сигнала ПЭП, формирование А-скана и передачу пакета с данными на ПК\", \"ID\": \"Receiver2Enable\", \"Max\": 1, \"Min\": 0, \"Name\": \"Разрешить работу приемника\", \"Row\": 4, \"Unit\": \"\" }, { \"Desc\": \"Номер ПЭП (с 9 по 16) подключенный ко входу приемника № 2\", \"ID\": \"Receiver2Multiplexer\", \"Max\": 16, \"Min\": 9, \"Name\": \"№ ПЭП (с 9 по 16) подключенный к приемнику №2\", \"Row\": 5, \"Unit\": \"\" }, { \"Desc\": \"Задержка начала развертки сигнала приемника №2 в такте\", \"ID\": \"ScanDelay2\", \"Max\": 200, \"Min\": 0, \"Name\": \"Задержка развертки приемника №2\", \"Row\": 6, \"Unit\": \"мкс\" }, { \"Desc\": \"Длительность записи сигнала приемника №2 в такте\", \"ID\": \"ScanDuration2\", \"Max\": 80, \"Min\": 1, \"Name\": \"Длительность развертки приемника №2\", \"Row\": 7, \"Unit\": \"мкс\" }, { \"Desc\": \"Коэффициент усиления предварительного усилителя приемника сигналов ПЭП №2\", \"ID\": \"Receiver2StaticGain\", \"Max\": 100, \"Min\": -100, \"Name\": \"Коэффициент усиления приемника №2\", \"Row\": 8, \"Unit\": \"дБ\" }, { \"Desc\": \"Выходное значение ЦАП №2\", \"ID\": \"Receiver2StaticGain\", \"Max\": 1023, \"Min\": 0, \"Name\": \"Выходное значение ЦАП №1 управляющий коэффициентом усиления приемника №2\", \"Row\": 9, \"Unit\": \"отсчет\" } ], \"Type\": \"Float\" }, { \"Num\": 2, \"Access\": \"ro\", \"ColumnCount\": 2, \"DataType\": \"float\", \"FormatStr\": \"%g\", \"ID\": \"RAWADCData\", \"Name\": \"Данные АЦП\", \"NeedParamPrepare\": true, \"RowCount\": 1, \"Columns\": [ { \"Column\": 0, \"Name\": \"Ось времени\", \"Type\": \"Regular\" }, { \"Column\": 1, \"Name\": \"Данные АЦП\", \"Type\": \"Regular\" } ] }, { \"Num\": 3, \"Access\": \"rw\", \"ColumnCount\": 10, \"NeedParamPrepare\": false, \"Columns\": [ { \"Column\": 0, \"Name\": \"0\" }, { \"Column\": 1, \"Name\": \"1\" }, { \"Column\": 2, \"Name\": \"2\" }, { \"Column\": 3, \"Name\": \"3\" }, { \"Column\": 4, \"Name\": \"4\" }, { \"Column\": 5, \"Name\": \"5\" }, { \"Column\": 6, \"Name\": \"6\" }, { \"Column\": 7, \"Name\": \"7\" }, { \"Column\": 8, \"Name\": \"8\" }, { \"Column\": 9, \"Name\": \"9\" } ], \"DataType\": \"float\", \"FormatStr\": \"%g\", \"ID\": \"CorPulseDurationP\", \"Name\": \"CorPulseDurationP\", \"RowCount\": 11, \"Desc\": \"Коррекция PulseDurationP\", \"Rows\": [ { \"ID\": \"PulseDuration\", \"Name\": \"PulseDuration / 10 [tick]\", \"Row\": 0 }, { \"ID\": \"CorPulseDurationP20V\", \"Name\": \"CorPulseDurationP20V\", \"Row\": 1 }, { \"ID\": \"CorPulseDurationP40V\", \"Name\": \"CorPulseDurationP40V\", \"Row\": 2 }, { \"ID\": \"CorPulseDurationP60V\", \"Name\": \"CorPulseDurationP60V\", \"Row\": 3 }, { \"ID\": \"CorPulseDurationP80V\", \"Name\": \"CorPulseDurationP80V\", \"Row\": 4 }, { \"ID\": \"CorPulseDurationP100V\", \"Name\": \"CorPulseDurationP100V\", \"Row\": 5 }, { \"ID\": \"CorPulseDurationP120V\", \"Name\": \"CorPulseDurationP120V\", \"Row\": 6 }, { \"ID\": \"CorPulseDurationP140V\", \"Name\": \"CorPulseDurationP140V\", \"Row\": 7 }, { \"ID\": \"CorPulseDurationP160V\", \"Name\": \"CorPulseDurationP160V\", \"Row\": 8 }, { \"ID\": \"CorPulseDurationP180V\", \"Name\": \"CorPulseDurationP180V\", \"Row\": 9 }, { \"ID\": \"CorPulseDurationP200V\", \"Name\": \"CorPulseDurationP200V\", \"Row\": 10 } ], \"Type\": \"Float\" }, { \"Num\": 4, \"Access\": \"rw\", \"ColumnCount\": 10, \"NeedParamPrepare\": false, \"Columns\": [ { \"Column\": 0, \"Name\": \"0\" }, { \"Column\": 1, \"Name\": \"1\" }, { \"Column\": 2, \"Name\": \"2\" }, { \"Column\": 3, \"Name\": \"3\" }, { \"Column\": 4, \"Name\": \"4\" }, { \"Column\": 5, \"Name\": \"5\" }, { \"Column\": 6, \"Name\": \"6\" }, { \"Column\": 7, \"Name\": \"7\" }, { \"Column\": 8, \"Name\": \"8\" }, { \"Column\": 9, \"Name\": \"9\" } ], \"DataType\": \"float\", \"FormatStr\": \"%g\", \"ID\": \"CorPulseDurationN\", \"Name\": \"CorPulseDurationN\", \"RowCount\": 11, \"Desc\": \"Коррекция PulseDurationN\", \"Rows\": [ { \"ID\": \"PulseDuration\", \"Name\": \"PulseDuration / 10 [tick]\", \"Row\": 0 }, { \"ID\": \"CorPulseDurationN20V\", \"Name\": \"CorPulseDurationN20V\", \"Row\": 1 }, { \"ID\": \"CorPulseDurationN40V\", \"Name\": \"CorPulseDurationN40V\", \"Row\": 2 }, { \"ID\": \"CorPulseDurationN60V\", \"Name\": \"CorPulseDurationN60V\", \"Row\": 3 }, { \"ID\": \"CorPulseDurationN80V\", \"Name\": \"CorPulseDurationN80V\", \"Row\": 4 }, { \"ID\": \"CorPulseDurationN100V\", \"Name\": \"CorPulseDurationN100V\", \"Row\": 5 }, { \"ID\": \"CorPulseDurationN120V\", \"Name\": \"CorPulseDurationN120V\", \"Row\": 6 }, { \"ID\": \"CorPulseDurationN140V\", \"Name\": \"CorPulseDurationN140V\", \"Row\": 7 }, { \"ID\": \"CorPulseDurationN160V\", \"Name\": \"CorPulseDurationN160V\", \"Row\": 8 }, { \"ID\": \"CorPulseDurationN180V\", \"Name\": \"CorPulseDurationN180V\", \"Row\": 9 }, { \"ID\": \"CorPulseDurationN200V\", \"Name\": \"CorPulseDurationN200V\", \"Row\": 10 } ], \"Type\": \"Float\" }, { \"Num\": 5, \"Access\": \"rw\", \"ColumnCount\": 1, \"NeedParamPrepare\": false, \"Columns\": [ { \"Column\": 0, \"Name\": \"0\" } ], \"DataType\": \"float\", \"FormatStr\": \"%g\", \"ID\": \"GainOffsetCor\", \"Name\": \"GainOffsetCor\", \"Desc\": \"Коррекция усиления по каналам\", \"RowCount\": 16, \"Rows\": [ { \"ID\": \"GOffset1\", \"Name\": \"GOffsetCh1\", \"Row\": 0 }, { \"ID\": \"GOffset2\", \"Name\": \"GOffsetCh2\", \"Row\": 1 }, { \"ID\": \"GOffset3\", \"Name\": \"GOffsetCh3\", \"Row\": 2 }, { \"ID\": \"GOffset4\", \"Name\": \"GOffsetCh4\", \"Row\": 3 }, { \"ID\": \"GOffset5\", \"Name\": \"GOffsetCh5\", \"Row\": 4 }, { \"ID\": \"GOffset6\", \"Name\": \"GOffsetCh6\", \"Row\": 5 }, { \"ID\": \"GOffset7\", \"Name\": \"GOffsetCh7\", \"Row\": 6 }, { \"ID\": \"GOffset8\", \"Name\": \"GOffsetCh8\", \"Row\": 7 }, { \"ID\": \"GOffset9\", \"Name\": \"GOffsetCh9\", \"Row\": 8 }, { \"ID\": \"GOffset10\", \"Name\": \"GOffsetCh10\", \"Row\": 9 }, { \"ID\": \"GOffset11\", \"Name\": \"GOffsetCh11\", \"Row\": 10 }, { \"ID\": \"GOffset12\", \"Name\": \"GOffsetCh12\", \"Row\": 11 }, { \"ID\": \"GOffset13\", \"Name\": \"GOffsetCh13\", \"Row\": 12 }, { \"ID\": \"GOffset14\", \"Name\": \"GOffsetCh14\", \"Row\": 13 }, { \"ID\": \"GOffset15\", \"Name\": \"GOffsetCh15\", \"Row\": 14 }, { \"ID\": \"GOffset16\", \"Name\": \"GOffsetCh16\", \"Row\": 15 } ], \"Type\": \"Float\" }, { \"Num\": 6, \"Access\": \"rw\", \"ColumnCount\": 2, \"NeedParamPrepare\": false, \"Columns\": [ { \"Column\": 0, \"Name\": \"GainCor_PL0\" }, { \"Column\": 1, \"Name\": \"GainCor_PL1\" } ], \"DataType\": \"float\", \"FormatStr\": \"%g\", \"ID\": \"GainCor\", \"Name\": \"GainCor\", \"Desc\": \"Коррекция усиления взависимости от установленного усиления\", \"RowCount\": 80, \"Rows\": [ ], \"Type\": \"Float\" }, { \"Num\": 7, \"Access\": \"rw\", \"ColumnCount\": 2, \"NeedParamPrepare\": false, \"Columns\": [ { \"Column\": 0, \"Name\": \"PAB0_SellHVFine\" }, { \"Column\": 1, \"Name\": \"PAB1_SellHVFine\" } ], \"DataType\": \"float\", \"FormatStr\": \"%g\", \"ID\": \"SellHVFine\", \"Name\": \"SellHVFine\", \"Desc\": \"Коррекция амплитуды возбуждения\", \"RowCount\": 10, \"Rows\": [ ], \"Type\": \"Float\" }, { \"Num\": 8, \"Access\": \"rw\", \"ColumnCount\": 2, \"NeedParamPrepare\": false, \"Columns\": [ { \"Column\": 0, \"Name\": \"PAB0_CorTransistor\" }, { \"Column\": 1, \"Name\": \"PAB1_CorTransistor\" } ], \"DataType\": \"float\", \"FormatStr\": \"%g\", \"ID\": \"PABx_CorTransistor\", \"Name\": \"PABx_CorTransistor\", \"Desc\": \"Коррекция времени возбуждения\", \"RowCount\": 8, \"Rows\": [ ], \"Type\": \"Float\" } ], \"UART\": [ { \"Name\": \"115200\", \"Value\": 4 } ] }"
  out "ArrayInt":i32[](array[numeric])
  in  "TblInt":string[][](table) caption="Параметры типа \"Int\""
  out "ArrayFloat":sgl[](array[numeric])
  out "1D Array 3":string[](array[string])=["\"Разрешить работу ГИ №1\"", "\"№ ПЭП (с 1 по 8) подключенный к ГИ №1\"", "\"Задержка импульса ГИ №1\"", "\"Длительность импульса ГИ\"", "\"Разрешить работу приемника\"", "\"№ ПЭП (с 1 по 8) подключенный к приемнику №1\"", "\"Задержка развертки приемника №1\"", "\"Длительность развертки приемника №1\"", "\"Коэффициент усиления приемника №1\"", "\"Выходное значение ЦАП №1 управляющий коэффициентом усиления приемника №1\"", "", "", "", "", "", ""]
  in  "TblParam1":sgl[][](array[numeric])
  in  "TblParam0":sgl[][](array[numeric])
  out "TblTelem":string[][](table)=[["1", "Core uptime", "11382.9", "s"], ["2", "FPGA №1 uptime", "11385.0", "s"], ["3", "FPGA №2 uptime", "11385.0", "s"], ["4", "TelStatusHF_EU", "0", ""], ["5", "Энкодер №1", "0", "мкм"], ["6", "Счетчик импыльсов", "1", "мкм"], ["7", "EncoderParam1", "2", "мкм"], ["8", "EncoderParam2", "3", "мкм"], ["9", "Tel33VDMON_G_min", "3.383", "В"], ["10", "Tel33VDMON_G_avg", "3.200", "В"], ["11", "Tel33VDMON_G_max", "3.416", "В"], ["12", "TelPMD2TempSensor", "34.8", "°C"], ["13", "TelPMD2TempDS18B20", "40.8", "°C"], ["14", "TelPMD6TempSensor", "34.0", "°C"], ["15", "TelPMD6TempDS18B20", "33.2", "°C"], ["16", "rb0_TempSensor", "27.5", "°C"], ["17", "rb1_TempSensor", "30.4", "°C"], ["18", "afe0_TempSensor", "32.8", "°C"], ["19", "afe0_TempDS18B20", "33.4", "°C"], ["20", "afe1_TempSensor", "33.0", "°C"], ["21", "afe1_TempDS18B20", "36.2", "°C"], ["22", "pab0_TempSensor", "34.3", "°C"], ["23", "pab0_TempDS18B20", "37.8", "°C"], ["24", "pab1_TempSensor", "28.2", "°C"], ["25", "pab1_TempDS18B20", "35.0", "°C"], ["26", "TelPMD2CInMin", "2.160", "A"], ["27", "TelPMD2CInAVG", "2.197", "A"], ["28", "TelPMD2CInMax", "2.236", "A"], ["29", "TelPMD2VInMin", "10.795", "V"], ["30", "TelPMD2VInAVG", "10.840", "V"], ["31", "TelPMD2VInMax", "10.859", "V"], ["32", "TelPMD2PInMin", "23.389", "W"], ["33", "TelPMD2PInAVG", "23.798", "W"], ["34", "TelPMD2PInMax", "24.198", "W"], ["35", "TelPMD2ConvFreq", "124994", "Hz"], ["36", "TelPMD6Vp220VMin", "223.956", "V"], ["37", "TelPMD6Vp220VAVG", "224.711", "V"], ["38", "TelPMD6Vp220VMax", "225.022", "V"], ["39", "TelPMD6Vp8VMin", "8.529", "V"], ["40", "TelPMD6Vp8VAVG", "8.553", "V"], ["41", "TelPMD6Vp8VMax", "8.568", "V"], ["42", "TelPMD6Vp5VMin", "4.998", "V"], ["43", "TelPMD6Vp5VAVG", "5.006", "V"], ["44", "TelPMD6Vp5VMax", "5.010", "V"], ["45", "TelPMD6Vp20VMin", "18.547", "V"], ["46", "TelPMD6Vp20VAVG", "18.593", "V"], ["47", "TelPMD6Vp20VMax", "18.623", "V"], ["48", "TelPMD6Vn8VMin", "-8.796", "V"], ["49", "TelPMD6Vn8VAVG", "-8.783", "V"], ["50", "TelPMD6Vn8VMax", "-8.762", "V"], ["51", "TelPMD6Vn20VMin", "-20.981", "V"], ["52", "TelPMD6Vn20VAVG", "-20.949", "V"], ["53", "TelPMD6Vn20VMax", "-20.906", "V"], ["54", "rb0_p_1v2d_G_min", "1.269", "V"], ["55", "rb0_p_1v2d_G_avg", "1.271", "V"], ["56", "rb0_p_1v2d_G_max", "1.272", "V"], ["57", "rb0_p_1v8a_G_min", "1.837", "V"], ["58", "rb0_p_1v8a_G_avg", "1.840", "V"], ["59", "rb0_p_1v8a_G_max", "1.843", "V"], ["60", "rb0_p_3v3d_G_min", "3.307", "V"], ["61", "rb0_p_3v3d_G_avg", "3.314", "V"], ["62", "rb0_p_3v3d_G_max", "3.319", "V"], ["63", "rb0_p_5va_G_min", "4.963", "V"], ["64", "rb0_p_5va_G_avg", "4.973", "V"], ["65", "rb0_p_5va_G_max", "4.979", "V"], ["66", "rb1_p_1v2d_G_min", "1.277", "V"], ["67", "rb1_p_1v2d_G_avg", "1.280", "V"], ["68", "rb1_p_1v2d_G_max", "1.282", "V"], ["69", "rb1_p_1v8a_G_min", "1.811", "V"], ["70", "rb1_p_1v8a_G_avg", "1.814", "V"], ["71", "rb1_p_1v8a_G_max", "1.816", "V"], ["72", "rb1_p_3v3d_G_min", "3.309", "V"], ["73", "rb1_p_3v3d_G_avg", "3.314", "V"], ["74", "rb1_p_3v3d_G_max", "3.319", "V"], ["75", "rb1_p_5va_G_min", "4.989", "V"], ["76", "rb1_p_5va_G_avg", "4.995", "V"], ["77", "rb1_p_5va_G_max", "5.000", "V"], ["78", "afe0_p_20v_G_min", "18.510", "V"], ["79", "afe0_p_20v_G_avg", "18.541", "V"], ["80", "afe0_p_20v_G_max", "18.567", "V"], ["81", "afe0_p_8v_G_min", "8.539", "V"], ["82", "afe0_p_8v_G_avg", "8.554", "V"], ["83", "afe0_p_8v_G_max", "8.568", "V"], ["84", "afe0_p_3v3_G_min", "3.297", "V"], ["85", "afe0_p_3v3_G_avg", "3.304", "V"], ["86", "afe0_p_3v3_G_max", "3.309", "V"], ["87", "afe0_p_v_protection_G_min", "4.779", "В"], ["88", "afe0_p_v_protection_G_avg", "4.802", "В"], ["89", "afe0_p_v_protection_G_max", "4.815", "В"], ["90", "afe0_m_v_protection_G_min", "-5.142", "В"], ["91", "afe0_m_v_protection_G_avg", "-5.128", "В"], ["92", "afe0_m_v_protection_G_max", "-5.108", "В"], ["93", "afe0_p_5va_G_min", "-5.172", "V"], ["94", "afe0_p_5va_G_avg", "-5.158", "V"], ["95", "afe0_p_5va_G_max", "-5.142", "V"], ["96", "afe0_m_5va_G_min", "4.876", "V"], ["97", "afe0_m_5va_G_avg", "4.887", "V"], ["98", "afe0_m_5va_G_max", "4.898", "V"], ["99", "afe1_p_20v_G_min", "18.599", "V"], ["100", "afe1_p_20v_G_avg", "18.625", "V"], ["101", "afe1_p_20v_G_max", "18.656", "V"], ["102", "afe1_p_8v_G_min", "8.539", "V"], ["103", "afe1_p_8v_G_avg", "8.551", "V"], ["104", "afe1_p_8v_G_max", "8.568", "V"], ["105", "afe1_p_3v3_G_min", "3.285", "V"], ["106", "afe1_p_3v3_G_avg", "3.290", "V"], ["107", "afe1_p_3v3_G_max", "3.295", "V"], ["108", "afe1_p_v_protection_G_min", "4.797", "В"], ["109", "afe1_p_v_protection_G_avg", "4.820", "В"], ["110", "afe1_p_v_protection_G_max", "4.828", "В"], ["111", "afe1_m_v_protection_G_min", "-5.187", "В"], ["112", "afe1_m_v_protection_G_avg", "-5.175", "В"], ["113", "afe1_m_v_protection_G_max", "-5.162", "В"], ["114", "afe1_p_5va_G_min", "-5.162", "V"], ["115", "afe1_p_5va_G_avg", "-5.147", "V"], ["116", "afe1_p_5va_G_max", "-5.128", "V"], ["117", "afe1_m_5va_G_min", "4.770", "V"], ["118", "afe1_m_5va_G_avg", "4.776", "V"], ["119", "afe1_m_5va_G_max", "4.782", "V"], ["120", "pab0_m_12v_G_min", "-11.801", "V"], ["121", "pab0_m_12v_G_avg", "-11.772", "V"], ["122", "pab0_m_12v_G_max", "-11.751", "V"], ["123", "pab0_m_20v_G_min", "-21.021", "V"], ["124", "pab0_m_20v_G_avg", "-20.964", "V"], ["125", "pab0_m_20v_G_max", "-20.947", "V"], ["126", "pab0_p_5v_G_min", "5.043", "V"], ["127", "pab0_p_5v_G_avg", "5.053", "V"], ["128", "pab0_p_5v_G_max", "5.065", "V"], ["129", "pab0_p_8v_G_min", "8.370", "V"], ["130", "pab0_p_8v_G_avg", "8.388", "V"], ["131", "pab0_p_8v_G_max", "8.400", "V"], ["132", "pab0_p_15v_G_min", "14.680", "V"], ["133", "pab0_p_15v_G_avg", "14.721", "V"], ["134", "pab0_p_15v_G_max", "14.751", "V"], ["135", "pab0_p_20v_G_min", "18.534", "V"], ["136", "pab0_p_20v_G_avg", "18.601", "V"], ["137", "pab0_p_20v_G_max", "18.623", "V"], ["138", "pab0_p_hv_G_min", "64.0", "V"], ["139", "pab0_p_hv_G_avg", "64.1", "V"], ["140", "pab0_p_hv_G_max", "64.3", "V"], ["141", "pab0_p_220v_G_min", "224.183", "V"], ["142", "pab0_p_220v_G_avg", "224.808", "V"], ["143", "pab0_p_220v_G_max", "225.074", "V"], ["144", "pab1_m_12v_G_min", "-11.665", "V"], ["145", "pab1_m_12v_G_avg", "-11.645", "V"], ["146", "pab1_m_12v_G_max", "-11.615", "V"], ["147", "pab1_m_20v_G_min", "-21.042", "V"], ["148", "pab1_m_20v_G_avg", "-20.971", "V"], ["149", "pab1_m_20v_G_max", "-20.933", "V"], ["150", "pab1_p_5v_G_min", "5.050", "V"], ["151", "pab1_p_5v_G_avg", "5.059", "V"], ["152", "pab1_p_5v_G_max", "5.068", "V"], ["153", "pab1_p_8v_G_min", "8.388", "V"], ["154", "pab1_p_8v_G_avg", "8.400", "V"], ["155", "pab1_p_8v_G_max", "8.415", "V"], ["156", "pab1_p_15v_G_min", "14.691", "V"], ["157", "pab1_p_15v_G_avg", "14.720", "V"], ["158", "pab1_p_15v_G_max", "14.746", "V"], ["159", "pab1_p_20v_G_min", "18.549", "V"], ["160", "pab1_p_20v_G_avg", "18.599", "V"], ["161", "pab1_p_20v_G_max", "18.638", "V"], ["162", "pab1_p_hv_G_min", "63.9", "V"], ["163", "pab1_p_hv_G_avg", "64.2", "V"], ["164", "pab1_p_hv_G_max", "64.4", "V"], ["165", "pab1_p_220v_G_min", "224.102", "V"], ["166", "pab1_p_220v_G_avg", "224.659", "V"], ["167", "pab1_p_220v_G_max", "224.993", "V"], ["168", "PM D2 Uptime", "03:10:08.000", ""], ["169", "PM D6 Uptime", "03:09:46.000", ""], ["170", "rb0 Uptime", "03:09:15.000", ""], ["171", "rb1 Uptime", "03:10:00.000", ""], ["172", "afe0 Uptime", "03:09:22.000", ""], ["173", "afe1 Uptime", "03:09:53.000", ""], ["174", "pab0 Uptime", "03:10:29.000", ""], ["175", "pab1 Uptime", "03:10:04.000", ""], ["176", "TelPMPassPacketCount", "22316", ""], ["177", "TelRB0PassPacketCount", "11135", ""], ["178", "TelRB1PassPacketCount", "11176", ""], ["179", "TelAFE0PassPacketCount", "11057", ""], ["180", "TelAFE1PassPacketCount", "11105", ""], ["181", "TelPAB0PassPacketCount", "11163", ""], ["182", "TelPAB1PassPacketCount", "11109", ""], ["183", "TelPMErrorPacketCount", "13", ""], ["184", "TelRB0ErrorPacketCount", "131", ""], ["185", "TelRB1ErrorPacketCount", "133", ""], ["186", "TelAFE0ErrorPacketCount", "185", ""], ["187", "TelAFE1ErrorPacketCount", "174", ""], ["188", "TelPAB0ErrorPacketCount", "149", ""], ["189", "TelPAB1ErrorPacketCount", "173", ""], ["190", "Frame Format Version", "0", ""], ["191", "N cycle", "0", ""], ["192", "N tick", "1", ""], ["193", "Global Time 1", "1138288", "Unix time"], ["194", "Global Time 2", "0", ""], ["195", "N chanel", "0", ""], ["196", "Scan Duration", "0", "пар семплов"], ["197", "CRC8", "0", ""], ["198", "CRC8 расчетный", "0", ""], ["199", "Scan Delay", "0", "отчет"], ["200", "Mux RX", "0", ""], ["201", "Mux TX", "0", ""], ["202", "Encoders Param 1", "0", ""], ["203", "Encoders Param 2", "0", ""], ["204", "Lose Packet", "0", ""], ["205", "Sample Interval", "0.000000", "с"], ["206", "Gain Coeff", "0.00", "дБ"], ["207", "Packet Counter", "0", ""], ["208", "Encoder1CurrData_PL0", "0", ""], ["209", "Encoder1CurrData_PL1", "0", ""], ["210", "Encoder2CurrData_PL0", "0", ""], ["211", "Encoder2CurrData_PL1", "0", ""], ["212", "PulseCurrData_PL0", "0", ""], ["213", "PulseCurrData_PL1", "0", ""], ["214", "NumOfRuns_PL0", "994875", ""], ["215", "NumOfRuns_PL1", "994870", ""], ["216", "Encoder1ScalingFactor_PL0", "1", ""], ["217", "TelRAMTestCompletionPercentage", "0.00", ""], ["218", "NumberOfApplicationLaunches", "82", ""], ["219", "TotalOperatingTime [min]", "3622", ""], ["220", "NumberOfFileRecords", "0", ""]] caption="Телеметрия"
  in  "LogoString":string
  out "LogoStop":bool
  in  "About_prg":T11={"Версия:"="", "Наименование ПО:"="SNK3.exe", "Год выпуска:"="2026", "Производитель:"="АО \"НИКИЭТ\"", "MD5"="", "Наименование ПО полное:"="Дефектоскоп ультразвуковой многоканальный акустический (ДУМА-16)", "Build"=""}
  in  "OptPACKPL1":T12={"MagicWordStr"="xV4\u0012", "Header size"=56, "Проверка CRC8"=TRUE, "Проверка конца пакета"=TRUE, "GainCompens"=FALSE, "Неотбрасывать BadEnd пакеты"=FALSE, "Неотбрасывать BadCRC пакеты"=FALSE, "Привести к 1"=FALSE, "GainCoef"=FALSE, "K_scale"=1.0, "ScaleOrdinate"=enum."Вольты"} {"K_scale" format="%_6g"}
  in  "OptPACKPL0":T12={"MagicWordStr"="xV4\u0012", "Header size"=56, "Проверка CRC8"=TRUE, "Проверка конца пакета"=TRUE, "GainCompens"=FALSE, "Неотбрасывать BadEnd пакеты"=FALSE, "Неотбрасывать BadCRC пакеты"=FALSE, "Привести к 1"=FALSE, "GainCoef"=FALSE, "K_scale"=1.0, "ScaleOrdinate"=enum."Вольты"} {"K_scale" format="%_6g"}
  in  "Ind":bool=TRUE
  out "UNDT_meas":string[][](table)=[["Частота, Гц", "1", "-", "-"], ["СКЗ, В", "1", "-", "-"], ["Амплитуда, В", "1", "-", "-"], ["Амплитуда, дБмкВ", "1", "-", "-"], ["Датчик пути 1, мм", "1", "-", "-"], ["Датчик пути 2, мм", "1", "-", "-"], ["Время, сек", "1", "-", "-"]]
  in  "AScanOscNum":u8
  out "AScanOsc":dbl[](array[numeric])
  out "MeasOut":T13[](array[typedef])=[{"FFT amplitude"=0.0909690140521737, "amplitude"=0.0, "RMS"=0.0, "detected frequency"=4999876.6919549145, "way sensor 1"=0.0, "way sensor 2"=-0.30000000000000000001, "detected frequency 2"=0.0, "time trig"=1e-05, "time trig 2"=0.0, "DC"=0.0, "trigger detected?"=FALSE, "FFT amplitude mean"=0.0}, {"FFT amplitude"=0.00043858891909434795, "amplitude"=0.0, "RMS"=0.0, "detected frequency"=3529512.357106555, "way sensor 1"=-0.2, "way sensor 2"=-0.30000000000000000001, "detected frequency 2"=0.0, "time trig"=0.0, "time trig 2"=0.0, "DC"=0.0, "trigger detected?"=FALSE, "FFT amplitude mean"=0.0}] {"FFT amplitude mean" format="%.2p"; "DC" format="%0.2p"; "time trig 2" format="%0.2p"; "time trig" format="%0.2p"; "detected frequency 2" format="%.2p"; "way sensor 2" format="%.2p"; "way sensor 1" format="%.2p"; "detected frequency" format="%.2p"; "RMS" format="%0.2p"; "amplitude" format="%.2p"; "FFT amplitude" format="%.2p"}
  out "Spectr_save":cluster{"f0":dbl, "df":dbl, "magnitude":dbl[]}[](array[cluster])
  out "GUI_Tick1Ctl":refnum<vi>[](array[refnum])
  out "GUI_Tick0Ctl":refnum<vi>[](array[refnum])
  out "GUI_AllControl":refnum<vi>[](array[refnum])
  out "#el_queue GUI":i32
  out "elementsGUI":string[](array[string])
  out "elementGUI":string
  out "DbgArray":u32[](array[numeric])
  in  "Stop":bool
  out "cycle1":bool
  out "cycle0":bool
  out "cycle2":bool
  out "cycle3":bool
  in  "Log_path":path
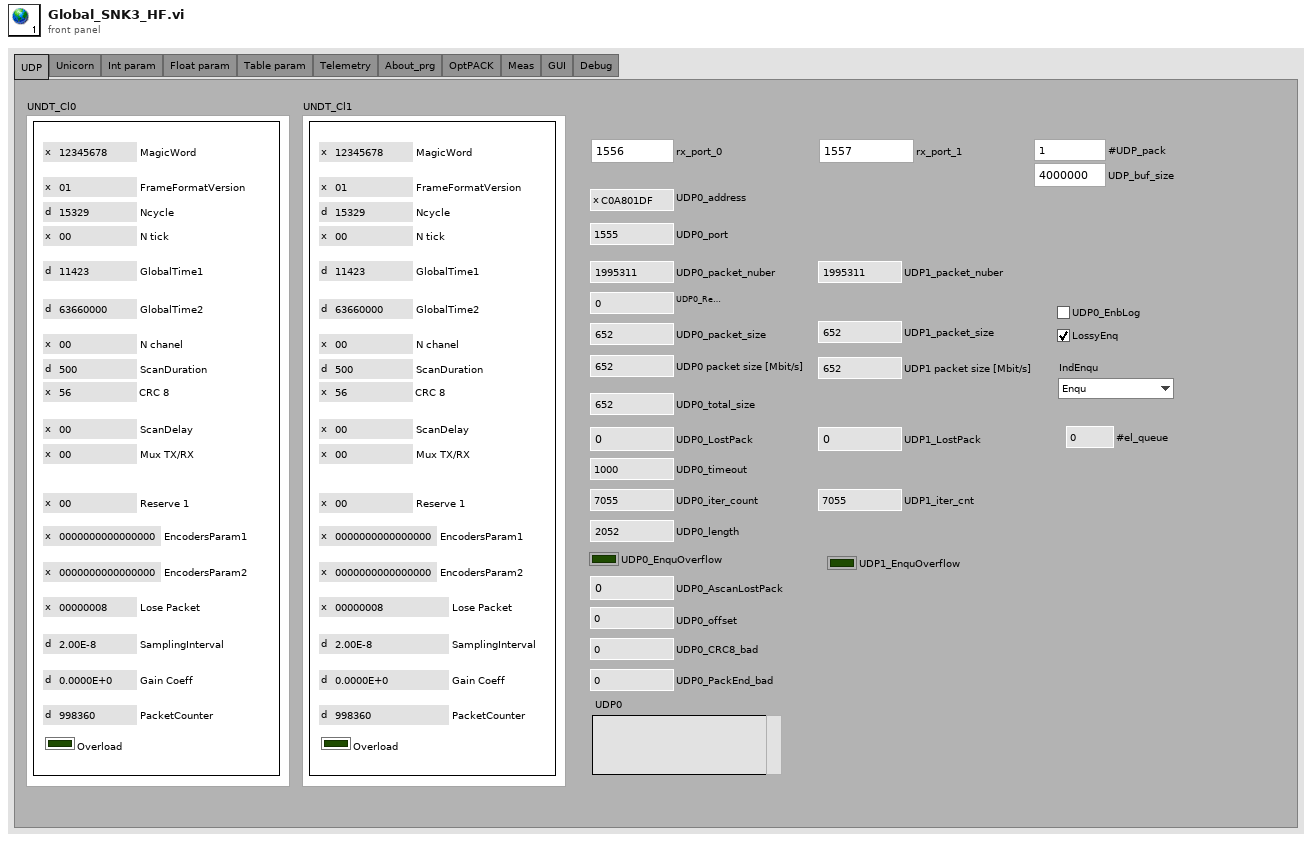
[diagram p1: front panel]
types:
  T1 = enum32{"UDP", "Unicorn", "Int param", "Float param", "Table param", "Telemetry", "About_prg", "OptPACK", "Meas", "GUI", "Debug"}
  T2 = typedef "UNDT_ClusterPackRevers (Type).ctl" = cluster{"PacketCounter":u32, "Gain Coeff":sgl, "SamplingInterval":sgl, "Lose Packet":u32, "EncodersParam2":u64, "EncodersParam1":u64, "Reserve 1":u8, "Mux TX/RX":u8, "ScanDelay":u16, "CRC 8":u8, "ScanDuration":u16, "N chanel":u8, "GlobalTime2":u32, "GlobalTime1":u32, "N tick":u8, "Ncycle":u16, "FrameFormatVersion":u8, "MagicWord":u32, "Overload":bool}
  T3 = typedef "LV_Unicorn.lvlib/AnswerUDP.ctl" = cluster{"IP":string, "Port":u16, "DataVersion":u16, "ModbusAddress":i32, "type_version":string, "Description":string, "Serial":string, "ServerPort":u16}
  T4 = typedef "LV_Unicorn.lvlib/unicorn_Param.ctl" = cluster{"conParam":T5, "Param":T6}
  T5 = typedef "LV_Unicorn.lvlib/unicorn_conn.ctl" = cluster{"ReadIntParam":bool, "ReadDescrParam":bool, "ReadFloatParam":bool, "debug":bool, "ReadJSON":bool, "IP_address":string, "N_attempts":i32, "type_con":enum16{"Serial", "TCP"}, "MB_address":i32, "VISA":refnum<visa-resource-name>, "connection ID":refnum<k5>, "nameDevices":string, "timeout":i32, "port":u16, "type_version":string, "baud_rate":u32, "VersionControl":bool, "TCP_conn":bool, "WindowSize":i32}
  T6 = typedef "LV_Unicorn.lvlib/unicorn_JSON.ctl" = cluster{"NumParam":cluster{"NTelem":i32, "NInt":i32, "NFloat":i32, "NTable":i32}, "ParamInt":T7, "Telemetry":T8, "Table":T9, "ParamFloat":T10}
  T7 = typedef "LV_Unicorn.lvlib/unicorn_ParamInt.ctl" = cluster{"ID":string, "Num":i32, "Name":string, "Type":string, "Enum":string, "Desc":string, "Unit":string, "Access":string, "FormatStr":string, "Min":i32, "Max":i32}[]
  T8 = typedef "LV_Unicorn.lvlib/unicorn_Telemetry.ctl" = cluster{"ID":string, "Num":i32, "Name":string, "Desc":string, "Unit":string, "FormatStr":string, "Min":i32, "Max":i32}[]
  T9 = typedef "LV_Unicorn.lvlib/unicorn_Table.ctl" = cluster{"Num":i32, "Access":string, "ColumnCount":i32, "NeedParamPrepare":bool, "Columns":cluster{"Column":i32, "Desc":string, "Name":string}[], "DataType":string, "FormatStr":string, "ID":string, "Name":string, "RowCount":i32, "Rows":cluster{"Desc":string, "ID":string, "Max":i32, "Min":i32, "Name":string, "Row":i32, "Unit":string}[], "Type":string}[]
  T10 = typedef "LV_Unicorn.lvlib/unicorn_ParamFloat.ctl" = cluster{"ID":string, "Num":i32, "Name":string, "Type":string, "Enum":string, "Desc":string, "Unit":string, "Access":string, "FormatStr":string, "Min":sgl, "Max":sgl}[]
  T11 = cluster{"Версия:":string, "Наименование ПО:":string, "Год выпуска:":string, "Производитель:":string, "MD5":string, "Наименование ПО полное:":string, "Build":string}
  T12 = typedef "OptionPACK5.ctl" = cluster{"MagicWordStr":string, "Header size":u32, "Проверка CRC8":bool, "Проверка конца пакета":bool, "GainCompens":bool, "Неотбрасывать BadEnd пакеты":bool, "Неотбрасывать BadCRC пакеты":bool, "Привести к 1":bool, "GainCoef":bool, "K_scale":dbl, "ScaleOrdinate":enum16{"Отсчеты АЦП (±32767)", "Проценты", "Вольты", "дБмкВ (отн. 1 мкВ)", "Отсчеты АЦП (±1)"}}
  T13 = typedef "MeasControl.ctl" = cluster{"FFT amplitude":dbl, "amplitude":dbl, "RMS":dbl, "detected frequency":dbl, "way sensor 1":ext, "way sensor 2":ext, "detected frequency 2":dbl, "time trig":dbl, "time trig 2":dbl, "DC":dbl, "trigger detected?":bool, "FFT amplitude mean":dbl}
diagram:
